vi "Save File DOE File Setup.vi"(0 "Filepath In":T10, 2 "Washer Controls In":T12={"Test Fixture Hardware"={"Power "={"Yokogawa"={"WT210"={"Sample Rate (1: 0.25s)"=1, "A Range (12: 20A)"=12, "V Range (6: 600V)"=4, "Power VISA Yokogawa WT210"="WT210"}, "WT500"={"Power VISA Yokogawa WT500"="WT500", "V Range (8: 1000V)"=0, "I Range (7: 40A)"=0, "Update Rate (3: 500ms)"=2}, "WT310_2"={"Sample Rate (1: 0.25s)"=1, "A Range (12: 20A)"=11, "V Range (6: 600V)"=4, "Power VISA Yokogawa WT310_2"="WT310_2"}, "WT310_3"={"Sample Rate (1: 0.25s)"=1, "A Range (12: 20A)"=11, "V Range (6: 600V)"=4, "Power VISA Yokogawa WT310_3"="WT310_3"}}, "Aplus"={"Aplus IP Address"="192.168.1.101", "Remote Port"=502, "Instrument"="APLUS", "Instr Driver Revision"="1.03.0053"}, "Power Limits"={"Crest Factor"={"Upper Limit"=1.49, "Lower Limit"=1.34}, "Harmonic Content"={"Uthd"=2.0}, "Voltage"={"% Error"=2.0}, "Stability"={"<1 Watt "={"Wattage"=1.0, "Slope (mW/H)"=10.0}, ">1 Watt"={"1%Power/Hour"=1.0}}}, "Nominal Voltage"=120, "Time Limit (s)"=10800.0, "Power Variation Limit (%)"=50.0, "Power Supply"={"Chroma 61605"="CHROMA", "Use Chroma?"=FALSE}}, "Weight Scale"={"Com Options"={"IND560Scale VISA"="IND560", "IP Address"="192.168.1.50", "Remote Port"=502, "Setra Scale VISA"="MW100", "GSE 350"="GSE350"}, "Select Scale"=""}, "Flow Rates"={"Laurel Cold IP Address"="", "Laurel Hot IP Address"="34972A_2", "Hot Water Laurel VISA"="LaurelMeter_Hot", "Cold Water Laurel VISA"="LaurelMeter_Cold", "Remote Port"=0, "Laurel Communication Type"="", "Meters To Collect (Hot Cold)"="", "HOT Laurel Reference"=refnum, "COLD Laurel Reference"=refnum}, "Analog Data"={"Agilent"={"Agilent 34972_1"="34972A_1", "Agilent 34972_2"="34972A_2", "Agilent 34972_3"="34972A_3", "Agilent 34972_4"="34972A_4", "Agilent 34972_5"="34972A_5", "Agilent 34972_6"="34972A_6", "Agilent Gain"=0.0, "TC Type (K,J,T)"="", "Instrument IDN?"="", "TC Channels-List"="", "Analog Channels-List"="", "Agilent Cluster Array"=[], "TC Channels-List 2"="", "Analog Channels-List 2"=""}, "Yokogawa"={"MW100"="MW100", "Intellifaucet"=FALSE}, "Select Analog"="", "TC Coefficients"={"TC Coefficients 1"=[], "TC Coefficients 2"=[], "TC Coefficients 3"=[], "TC Coefficients 4"=[], "TC Coefficients 5"=[], "TC Coefficients 6"=[], "TC Coefficients 7"=[]}, "NI Tasks (Dryer DOE)"=["TC Temps-Module 1", "TC Temps-Module 2", "TC Temps-Module 3", "TC Temps-Module 4", "TC Temps-Module 5", "Gas and Temp-Module 6", "AC_DC Events-Module 7"], "Laurel Analog"={"Laurel IP (Water Temp)"="", "Laurel IP (Pressure)"=""}}, "ITHX-Temp Humidity"={"IP Address 1"="", "Remote Port"=0, "IP Address 2"="", "IP Address 3"=""}, "Gas Meter COM Ports"={"Gas Meter 1"="COM3", "Gas Meter 2"="COM4", "Gas Meter 3"="COM5", "Gas Meter 4"="COM6", "Gas Meter 5"="COM7", "Gas Meter 6"="COM8"}, "Barometric Pressure"={"HEISE 901A"="HEISE", "Use Barometer?"=FALSE}}, "GEA2"={"Address"=35, "Source"=228, "Viper/Hawk"=0}, "DOE Capacity Measurments"={"Weight 1"=35.0, "Model Number 1"="", "Temp 1"=0.0, "Serial Number 1"="", "Lab Number 1"="", "Lab Number 2"="", "Serial Number 2"="", "Temp 2"=0.0, "Model Number 2"="", "Weight 2"=0.0, "Lab Number 3"="", "Serial Number 3"="", "Temp 3"=0.0, "Model Number 3"="", "Weight 3"=0.0, "Lab Number 4"="", "Serial Number 4"="", "Temp 4"=0.0, "Model Number 4"="", "Weight 4"=0.0, "Capacity Measurment Output String"=[]}, "Initialize.Washer In"={"Appliance Details"={"FileVersionInfo"={"FileVersion"="", "ProductName"="", "InternalName"="", "CompanyName"="", "LegalCopyright"="", "FileDescription"=""}, "Dishwasher Info"={"Open Cup Weight (gm):"=0.0, "Auto Cup Weight (gm):"=0.0, "Detergent-Dish:"="", "Inlet Temperature-Dish:"="", "Cycle Mode-Dish:"="", "Unit Control-Dish:"="", "Manufacturer-Dish:"=""}, "Washer Info"={"Hot Water Temperature (Fahrenheit):"="", "Cold Water Temperature (Fahrenheit):"="", "Capacity (cu.ft):"=0.0, "Initial Cloth Weight:"=0.0, "Cloth Lot:"=60, "Model Family:"="", "Program Name:"="", "Cycle Selection:"="", "Wash Temperature:"="", "Rinse Temperature:"="", "Load Size:"=""}, "File Name Output Array"=[], "Calibration Output Array"=[], "Appliance Common"={"Engineer:"="", "Model Number:"="", "Serial Number:"="", "Comments:"="", "Station ID:"="", "Technician:"="", "TR Number:"="", "Lab ID:"="", "Voltage:"="", "Water Pressure (PSI):"="", "Test Date:"="", "Computer Name:"="", "IP Address:"="", "Ambient RH:"="", "Frequency:"="", "Build:"="", "Filename:"="", "Test Type:"="", "Load Run #:"=17, "Ambient Temperature (F):"="", "File Path:"=path "", "Cycles Per Year"=0}, "Water Heater"={"Heating Mode:"=""}, "Dryer"={"Heat Setting:"="", "Washer Water Temperature (60 ± 5°F):"=7, "Water Hardness (PPM):"=7, "Dryness Setting:"="", "Dryer Type:"="", "Exhaust:"="", "Drying Cycle:"="", "Load Type:"="", "Nominal Load Weight"="", "Dryer Initial IMC Data"={"Measured IMC (lbs)"=100.0, "Actual Initial RMC (%)"=7.0, "RMC (Desired %)"=5.0, "Bone Dry Wt(lbs)"=60.0, "Tolerance(%)"=0.0, "Actual Final RMC (%)"=7.0, "CEF (lbf/kWh)"=0.0, "Minimum Weight (lbf)"=0.0, "Average Weight (lbf)"=0.0, "Maximum Weight (lbf)"=0.0, "Measured IMC In Range?"=FALSE, "Moisture Reduction Factor"=55.5, "Field Use Factor"=1.04, "Empty Dryer Cold Weigth"=0.0, "Energy Standard"=enum."D2-Automatic Dryer", "Weight Cloth (lbs)"=0.0, "Relative Moisture Content (%)"=0.0, "Relative Moisture Content - Avg (%)"=0.0}}}, "Display Data (RLT)"={"Status Color"=0, "Serial Number Display"="", "Cycle Count Display"=0, "Station Label Display"="", "Current Run Start Time Display"=0.0, "Board ID Display"="", "RPM Display"=0, "Current Display"=0.0, "Current Path Display"=path "", "Saving Display"=FALSE, "Unit Type Display"=enum."", "Total Time On Display"=0.0, "UI Button"=FALSE}}} {"Initialize.Washer In"."Display Data (RLT)"."Current Display" format="%.2f"; "Initialize.Washer In"."Display Data (RLT)"."Cycle Count Display" format="%04d"; "Initialize.Washer In"."Appliance Details"."Dryer"."Dryer Initial IMC Data"."Maximum Weight (lbf)" format="%03_6g"; "Initialize.Washer In"."Appliance Details"."Dryer"."Dryer Initial IMC Data"."Average Weight (lbf)" format="%03_6g"; "Initialize.Washer In"."Appliance Details"."Dryer"."Dryer Initial IMC Data"."Minimum Weight (lbf)" format="%03_6g"; "Initialize.Washer In"."Appliance Details"."Dryer"."Dryer Initial IMC Data"."CEF (lbf/kWh)" format="%03_6g"; "Initialize.Washer In"."Appliance Details"."Dryer"."Dryer Initial IMC Data"."Actual Final RMC (%)" format="%03_6g"; "Initialize.Washer In"."Appliance Details"."Dryer"."Dryer Initial IMC Data"."Tolerance(%)" format="%0#_6g"; "Initialize.Washer In"."Appliance Details"."Dryer"."Dryer Initial IMC Data"."Bone Dry Wt(lbs)" format="%03_6g"; "Initialize.Washer In"."Appliance Details"."Dryer"."Dryer Initial IMC Data"."RMC (Desired %)" format="%0#_6g"; "Initialize.Washer In"."Appliance Details"."Dryer"."Dryer Initial IMC Data"."Actual Initial RMC (%)" format="%03_6g"; "Initialize.Washer In"."Appliance Details"."Dryer"."Dryer Initial IMC Data"."Measured IMC (lbs)" format="%0#_6g"; "GEA2"."Address" format="%x"; "GEA2"."Source" format="%x"; "GEA2"."Viper/Hawk" items=["Viper", "Hawk"]; "Test Fixture Hardware"."Power"."Yokogawa"."WT310_3"."V Range (6: 600V)" items=["Auto", "15V", "30V", "60V", "150V", "300V", "600V"]; "Test Fixture Hardware"."Power"."Yokogawa"."WT310_3"."A Range (12: 20A)" items=["Auto", "5mA", "10mA", "20mA", "50mA", "100mA", "200mA", "0.5A", "1A", "2A", "5A", "10A", "20A", "50mV", "100mV", "200mV", "2.5V", "5V", "10V"]; "Test Fixture Hardware"."Power"."Yokogawa"."WT310_3"."Sample Rate (1: 0.25s)" items=["0.1s", "0.25s", "0.5s", "1s", "2s", "5s"]; "Test Fixture Hardware"."Power"."Yokogawa"."WT310_2"."V Range (6: 600V)" items=["Auto", "15V", "30V", "60V", "150V", "300V", "600V"]; "Test Fixture Hardware"."Power"."Yokogawa"."WT310_2"."A Range (12: 20A)" items=["Auto", "5mA", "10mA", "20mA", "50mA", "100mA", "200mA", "0.5A", "1A", "2A", "5A", "10A", "20A", "50mV", "100mV", "200mV", "2.5V", "5V", "10V"]; "Test Fixture Hardware"."Power"."Yokogawa"."WT310_2"."Sample Rate (1: 0.25s)" items=["0.1s", "0.25s", "0.5s", "1s", "2s", "5s"]; "Test Fixture Hardware"."Power"."Yokogawa"."WT500"."Update Rate (3: 500ms)" items=["-", "100ms", "200ms", "500ms", "1s", "2s", "5s"]; "Test Fixture Hardware"."Power"."Yokogawa"."WT500"."I Range (7: 40A)" items=["AUTO", "500 mA", "1 A", "2 A", "5 A", "10 A", "20 A", "40 A", "S-AUTO", "50 mV", "100 mV", "200 mV", "500 mV", "1 V", "2 V", "5 V", "10 V", "250 mA", "500 mA", "1 A", "2.5 A", "5 A", "10 A", "20 A", "25 mV", "50 mV", "100 mV", "250 mV", "500 mV", "1 V", "2.5 V", "5 V"]; "Test Fixture Hardware"."Power"."Yokogawa"."WT500"."V Range (8: 1000V)" items=["AUTO", "15", "30", "60", "100", "150", "300", "600", "1000", "7.5", "15", "30", "50", "75", "150", "300", "500"]; "Test Fixture Hardware"."Power"."Yokogawa"."WT210"."V Range (6: 600V)" items=["Auto", "15V", "30V", "60V", "150V", "300V", "600V"]; "Test Fixture Hardware"."Power"."Yokogawa"."WT210"."A Range (12: 20A)" items=["Auto", "5mA", "10mA", "20mA", "50mA", "100mA", "200mA", "0.5A", "1A", "2A", "5A", "10A", "20A", "50mV", "100mV", "200mV", "2.5V", "5V", "10V"]; "Test Fixture Hardware"."Power"."Yokogawa"."WT210"."Sample Rate (1: 0.25s)" items=["0.1s", "0.25s", "0.5s", "1s", "2s", "5s"]}, 3 "Station ID:":string(combo), 5 "error in (no error)":errorcluster, 6 "Config State":T8, 8 "LV Program":T9=enum."DOE Stand") -> (14 "Washer Controls Out":T12={"Test Fixture Hardware"={"Power "={"Yokogawa"={"WT210"={"Sample Rate (1: 0.25s)"=1, "A Range (12: 20A)"=12, "V Range (6: 600V)"=4, "Power VISA Yokogawa WT210"="WT210"}, "WT500"={"Power VISA Yokogawa WT500"="WT500", "V Range (8: 1000V)"=0, "I Range (7: 40A)"=0, "Update Rate (3: 500ms)"=2}, "WT310_2"={"Sample Rate (1: 0.25s)"=1, "A Range (12: 20A)"=11, "V Range (6: 600V)"=4, "Power VISA Yokogawa WT310_2"="WT310_2"}, "WT310_3"={"Sample Rate (1: 0.25s)"=1, "A Range (12: 20A)"=11, "V Range (6: 600V)"=4, "Power VISA Yokogawa WT310_3"="WT310_3"}}, "Aplus"={"Aplus IP Address"="192.168.1.101", "Remote Port"=502, "Instrument"="APLUS", "Instr Driver Revision"="1.03.0053"}, "Power Limits"={"Crest Factor"={"Upper Limit"=1.49, "Lower Limit"=1.34}, "Harmonic Content"={"Uthd"=2.0}, "Voltage"={"% Error"=2.0}, "Stability"={"<1 Watt "={"Wattage"=1.0, "Slope (mW/H)"=10.0}, ">1 Watt"={"1%Power/Hour"=1.0}}}, "Nominal Voltage"=120, "Time Limit (s)"=10800.0, "Power Variation Limit (%)"=50.0, "Power Supply"={"Chroma 61605"="CHROMA", "Use Chroma?"=FALSE}}, "Weight Scale"={"Com Options"={"IND560Scale VISA"="IND560", "IP Address"="192.168.1.50", "Remote Port"=502, "Setra Scale VISA"="SETRA", "GSE 350"="GSE350"}, "Select Scale"=""}, "Flow Rates"={"Laurel Cold IP Address"="", "Laurel Hot IP Address"="", "Hot Water Laurel VISA"="34972A_3", "Cold Water Laurel VISA"="MW100", "Remote Port"=0, "Laurel Communication Type"="", "Meters To Collect (Hot Cold)"="", "HOT Laurel Reference"=refnum, "COLD Laurel Reference"=refnum}, "Analog Data"={"Agilent"={"Agilent 34972_1"="34972A_1", "Agilent 34972_2"="34972A_2", "Agilent 34972_3"="34972A_3", "Agilent 34972_4"="34972A_3", "Agilent 34972_5"="34972A_3", "Agilent 34972_6"="34972A_3", "Agilent Gain"=0.0, "TC Type (K,J,T)"="", "Instrument IDN?"="", "TC Channels-List"="", "Analog Channels-List"="", "Agilent Cluster Array"=[], "TC Channels-List 2"="", "Analog Channels-List 2"=""}, "Yokogawa"={"MW100"="MW100", "Intellifaucet"=FALSE}, "Select Analog"="", "TC Coefficients"={"TC Coefficients 1"=[], "TC Coefficients 2"=[], "TC Coefficients 3"=[], "TC Coefficients 4"=[], "TC Coefficients 5"=[], "TC Coefficients 6"=[], "TC Coefficients 7"=[]}, "NI Tasks (Dryer DOE)"=["TC Temps-Module 1", "TC Temps-Module 2", "TC Temps-Module 3", "TC Temps-Module 4", "TC Temps-Module 5", "Gas and Temp-Module 6", "AC_DC Events-Module 7"], "Laurel Analog"={"Laurel IP (Water Temp)"="", "Laurel IP (Pressure)"=""}}, "ITHX-Temp Humidity"={"IP Address 1"="", "Remote Port"=0, "IP Address 2"="", "IP Address 3"=""}, "Gas Meter COM Ports"={"Gas Meter 1"="COM3", "Gas Meter 2"="COM4", "Gas Meter 3"="COM5", "Gas Meter 4"="COM6", "Gas Meter 5"="COM7", "Gas Meter 6"="COM8"}, "Barometric Pressure"={"HEISE 901A"="HEISE", "Use Barometer?"=FALSE}}, "GEA2"={"Address"=35, "Source"=228, "Viper/Hawk"=0}, "DOE Capacity Measurments"={"Weight 1"=35.0, "Model Number 1"="", "Temp 1"=0.0, "Serial Number 1"="", "Lab Number 1"="", "Lab Number 2"="", "Serial Number 2"="", "Temp 2"=0.0, "Model Number 2"="", "Weight 2"=0.0, "Lab Number 3"="", "Serial Number 3"="", "Temp 3"=0.0, "Model Number 3"="", "Weight 3"=0.0, "Lab Number 4"="", "Serial Number 4"="", "Temp 4"=0.0, "Model Number 4"="", "Weight 4"=0.0, "Capacity Measurment Output String"=[]}, "Initialize.Washer In"={"Appliance Details"={"FileVersionInfo"={"FileVersion"="", "ProductName"="", "InternalName"="", "CompanyName"="", "LegalCopyright"="", "FileDescription"=""}, "Dishwasher Info"={"Open Cup Weight (gm):"=0.0, "Auto Cup Weight (gm):"=0.0, "Detergent-Dish:"="", "Inlet Temperature-Dish:"="", "Cycle Mode-Dish:"="", "Unit Control-Dish:"="", "Manufacturer-Dish:"=""}, "Washer Info"={"Hot Water Temperature (Fahrenheit):"="", "Cold Water Temperature (Fahrenheit):"="", "Capacity (cu.ft):"=0.0, "Initial Cloth Weight:"=0.0, "Cloth Lot:"=60, "Model Family:"="", "Program Name:"="", "Cycle Selection:"="", "Wash Temperature:"="", "Rinse Temperature:"="", "Load Size:"=""}, "File Name Output Array"=[], "Calibration Output Array"=[], "Appliance Common"={"Engineer:"="", "Model Number:"="", "Serial Number:"="", "Comments:"="", "Station ID:"="", "Technician:"="", "TR Number:"="", "Lab ID:"="", "Voltage:"="", "Water Pressure (PSI):"="", "Test Date:"="", "Computer Name:"="", "IP Address:"="", "Ambient RH:"="", "Frequency:"="", "Build:"="", "Filename:"="", "Test Type:"="", "Load Run #:"=17, "Ambient Temperature (F):"="", "File Path:"=path "", "Cycles Per Year"=0}, "Water Heater"={"Heating Mode:"=""}, "Dryer"={"Heat Setting:"="", "Washer Water Temperature (60 ± 5°F):"=7, "Water Hardness (PPM):"=7, "Dryness Setting:"="", "Dryer Type:"="", "Exhaust:"="", "Drying Cycle:"="", "Load Type:"="", "Nominal Load Weight"="", "Dryer Initial IMC Data"={"Measured IMC (lbs)"=100.0, "Actual Initial RMC (%)"=7.0, "RMC (Desired %)"=5.0, "Bone Dry Wt(lbs)"=60.0, "Tolerance(%)"=0.0, "Actual Final RMC (%)"=7.0, "CEF (lbf/kWh)"=0.0, "Minimum Weight (lbf)"=0.0, "Average Weight (lbf)"=0.0, "Maximum Weight (lbf)"=0.0, "Measured IMC In Range?"=FALSE, "Moisture Reduction Factor"=55.5, "Field Use Factor"=1.04, "Empty Dryer Cold Weigth"=0.0, "Energy Standard"=enum."D2-Automatic Dryer", "Weight Cloth (lbs)"=0.0, "Relative Moisture Content (%)"=0.0, "Relative Moisture Content - Avg (%)"=0.0}}}, "Display Data (RLT)"={"Status Color"=0, "Serial Number Display"="", "Cycle Count Display"=0, "Station Label Display"="", "Current Run Start Time Display"=0.0, "Board ID Display"="", "RPM Display"=0, "Current Display"=0.0, "Current Path Display"=path "", "Saving Display"=FALSE, "Unit Type Display"=enum."", "Total Time On Display"=0.0, "UI Button"=FALSE}}} {"Initialize.Washer In"."Display Data (RLT)"."Current Display" format="%.2f"; "Initialize.Washer In"."Display Data (RLT)"."Cycle Count Display" format="%04d"; "Initialize.Washer In"."Appliance Details"."Dryer"."Dryer Initial IMC Data"."Maximum Weight (lbf)" format="%03_6g"; "Initialize.Washer In"."Appliance Details"."Dryer"."Dryer Initial IMC Data"."Average Weight (lbf)" format="%03_6g"; "Initialize.Washer In"."Appliance Details"."Dryer"."Dryer Initial IMC Data"."Minimum Weight (lbf)" format="%03_6g"; "Initialize.Washer In"."Appliance Details"."Dryer"."Dryer Initial IMC Data"."CEF (lbf/kWh)" format="%03_6g"; "Initialize.Washer In"."Appliance Details"."Dryer"."Dryer Initial IMC Data"."Actual Final RMC (%)" format="%03_6g"; "Initialize.Washer In"."Appliance Details"."Dryer"."Dryer Initial IMC Data"."Tolerance(%)" format="%0#_6g"; "Initialize.Washer In"."Appliance Details"."Dryer"."Dryer Initial IMC Data"."Bone Dry Wt(lbs)" format="%03_6g"; "Initialize.Washer In"."Appliance Details"."Dryer"."Dryer Initial IMC Data"."RMC (Desired %)" format="%0#_6g"; "Initialize.Washer In"."Appliance Details"."Dryer"."Dryer Initial IMC Data"."Actual Initial RMC (%)" format="%03_6g"; "Initialize.Washer In"."Appliance Details"."Dryer"."Dryer Initial IMC Data"."Measured IMC (lbs)" format="%0#_6g"; "GEA2"."Address" format="%x"; "GEA2"."Source" format="%x"; "GEA2"."Viper/Hawk" items=["Viper", "Hawk"]; "Test Fixture Hardware"."Power"."Yokogawa"."WT310_3"."V Range (6: 600V)" items=["Auto", "15V", "30V", "60V", "150V", "300V", "600V"]; "Test Fixture Hardware"."Power"."Yokogawa"."WT310_3"."A Range (12: 20A)" items=["Auto", "5mA", "10mA", "20mA", "50mA", "100mA", "200mA", "0.5A", "1A", "2A", "5A", "10A", "20A", "50mV", "100mV", "200mV", "2.5V", "5V", "10V"]; "Test Fixture Hardware"."Power"."Yokogawa"."WT310_3"."Sample Rate (1: 0.25s)" items=["0.1s", "0.25s", "0.5s", "1s", "2s", "5s"]; "Test Fixture Hardware"."Power"."Yokogawa"."WT310_2"."V Range (6: 600V)" items=["Auto", "15V", "30V", "60V", "150V", "300V", "600V"]; "Test Fixture Hardware"."Power"."Yokogawa"."WT310_2"."A Range (12: 20A)" items=["Auto", "5mA", "10mA", "20mA", "50mA", "100mA", "200mA", "0.5A", "1A", "2A", "5A", "10A", "20A", "50mV", "100mV", "200mV", "2.5V", "5V", "10V"]; "Test Fixture Hardware"."Power"."Yokogawa"."WT310_2"."Sample Rate (1: 0.25s)" items=["0.1s", "0.25s", "0.5s", "1s", "2s", "5s"]; "Test Fixture Hardware"."Power"."Yokogawa"."WT500"."Update Rate (3: 500ms)" items=["-", "100ms", "200ms", "500ms", "1s", "2s", "5s"]; "Test Fixture Hardware"."Power"."Yokogawa"."WT500"."I Range (7: 40A)" items=["AUTO", "500 mA", "1 A", "2 A", "5 A", "10 A", "20 A", "40 A", "S-AUTO", "50 mV", "100 mV", "200 mV", "500 mV", "1 V", "2 V", "5 V", "10 V", "250 mA", "500 mA", "1 A", "2.5 A", "5 A", "10 A", "20 A", "25 mV", "50 mV", "100 mV", "250 mV", "500 mV", "1 V", "2.5 V", "5 V"]; "Test Fixture Hardware"."Power"."Yokogawa"."WT500"."V Range (8: 1000V)" items=["AUTO", "15", "30", "60", "100", "150", "300", "600", "1000", "7.5", "15", "30", "50", "75", "150", "300", "500"]; "Test Fixture Hardware"."Power"."Yokogawa"."WT210"."V Range (6: 600V)" items=["Auto", "15V", "30V", "60V", "150V", "300V", "600V"]; "Test Fixture Hardware"."Power"."Yokogawa"."WT210"."A Range (12: 20A)" items=["Auto", "5mA", "10mA", "20mA", "50mA", "100mA", "200mA", "0.5A", "1A", "2A", "5A", "10A", "20A", "50mV", "100mV", "200mV", "2.5V", "5V", "10V"]; "Test Fixture Hardware"."Power"."Yokogawa"."WT210"."Sample Rate (1: 0.25s)" items=["0.1s", "0.25s", "0.5s", "1s", "2s", "5s"]}, 16 "Filepath Out":T10, 19 "error out":errorcluster)   [LabVIEW 2018, in "File Setup.lvlib"]
uses:
  File Setup.lvlib
  Custom Pallet Controls/Custom Pallet String.ctl
  Custom Pallet Controls/Custom Pallet Forward.ctl
  Type Definition/Save File DOE LabView Program.ctl
  Type Definition/Save File DOE File Path Control.ctl
  Type Definition/Save File DOE Data Save Filepaths.ctl
  Type Definition/Save File DOE Configuration State.ctl
  Type Definition/Save File HEWH Heating Control Mode.ctl
  Washer DOE/Type Definitions/DOE Main Control.ctl
  Washer DOE/Type Definitions/DOE Test Fixture Hardware.ctl
  Type Definitions/UTILITY Power Inputs Control.ctl
  Drivers/IND560 Scale Monitor/Type Definitions/IND560 Configuration.ctl
  Hybrid Water Heater/Type Definitions/HEWH Agilent Cluster.ctl
  Type Definitions/UTILITY TC Coefficients.ctl
  Drivers/Omega FMA-1600A Series Gas Flow Meter/Type Definitions/FMA1600A COM Ports.ctl
  Washer DOE/Configuration/GEA2.ctl
  Washer DOE/Type Definitions/DOE Capacity Measurments.ctl
  Public/Type Definitions/Save File Washer.ctl
  Type Definition/Save File DISH Dishwasher Details.ctl
  <vilib>/Platform/fileVersionInfo.llb/FileVersionInformation.ctl
  Washer DOE/Type Definitions/DOE Appliance Common.ctl
  Type Definition/DPT IMC Data.ctl
  Washer DOE/Type Definitions/DOE Dryer Standard.ctl
  Public/Type Definitions/Save File Appliance Display.ctl
  Public/Type Definitions/Save File Unit Type.ctl
  GEA2 Commands/HEWH/Type Definitions/GEA2 Commands.ctl
  Type Definition/Save File Drop Down Controls.ctl
  <vilib>/Utility/file.llb/Write To Spreadsheet File (string).vi
  LabVIEW GEA2 Toolkit v1.0.0.0/library/GEA2_Toolkit.lvlib
  Save File.lvlib
panel:
  in  "Read Previous":bool
  in  "Comments:":string
  in  "Program Tab":T1(tab)
  in  "Remove Button 23":bool
  in  "Add Button 23":bool
  in  "Ambient Temperature (F):":string(combo)
  in  "Get Serial Number":bool
  in  "Get Model Number":bool
  in  "Remove Button 17":bool
  in  "Add Button 17":bool
  in  "Lab ID:":string(combo)
  in  "Remove Button 1":bool
  in  "Add Button 1":bool
  in  "Remove Button 2":bool
  in  "Add Button 2":bool
  in  "Technician:":string(combo)
  in  "Remove Button 3":bool
  in  "Add Button 3":bool
  in  "Water Pressure (PSI):":string(combo)
  in  "Remove Button 4":bool
  in  "Add Button 4":bool
  in  "Ambient RH:":string(combo)
  in  "Remove Button 5":bool
  in  "Add Button 5":bool
  in  "Supply Voltage:":string(combo)
  in  "Remove Button 6":bool
  in  "Add Button 6":bool
  in  "Frequency:":string(combo)
  in  "Remove Button 7":bool
  in  "Add Button 7":bool
  in  "Build:":string(combo)
  in  "TR Number:":string(combo)
  in  "Remove Button 16":bool
  in  "Add Button 16":bool
  in  "Remove Button 12":bool
  in  "Add Button 12":bool
  in  "Test Type:":string(combo)
  in  "Load Run #:":i32
  in  "Model:":T2
  in  "Serial Number:":T2
  in  "Engineer:":T2
  in  "Cycles Per Year":u32=283
  in  "Remove Button 21":bool
  in  "Add Button 21":bool
  in  "Cycle Selection":string(combo)
  in  "Remove Button 18":bool
  in  "Add Button 18":bool
  in  "Wash Temperature":string(combo)
  in  "Remove Button 19":bool
  in  "Add Button 19":bool
  in  "Rinse Temperature":string(combo)
  in  "Remove Button 20":bool
  in  "Add Button 20":bool
  in  "Load Size":string(combo)
  in  "Remove Button 9":bool
  in  "Add Button 9":bool
  in  "Cold Water Temperature (Fahrenheit)":string(combo)
  in  "Program Name":string(combo)
  in  "Model Family":string(combo)
  in  "Cloth Lot:":i32
  in  "Initial Cloth Weight:":dbl
  in  "Capacity (cu.ft)":dbl
  in  "Hot Water Temperature (Fahrenheit)":string(combo)
  in  "Remove Button 8":bool
  in  "Add Button 8":bool
  in  "Unit Type Display":T3
  in  "Remove Button 15":bool
  in  "Add Button 15":bool
  in  "Detergent-Dish:":string(combo)
  in  "Remove Button 14":bool
  in  "Add Button 14":bool
  in  "Inlet Temperature-Dish:":string(combo)
  in  "Remove Button 13":bool
  in  "Add Button 13":bool
  in  "Cycle Mode-Dish:":string(combo)
  in  "Remove Button 11":bool
  in  "Add Button 11":bool
  in  "Unit Control-Dish:":string(combo)
  in  "Manufacturer-Dish:":string(combo)
  in  "Remove Button 10":bool
  in  "Add Button 10":bool
  in  "Auto Cup Weight (gm):":dbl
  in  "Open Cup Weight (gm):":dbl
  in  "Heating Mode":T4
  in  "Remove Button 22":bool
  in  "Add Button 22":bool
  in  "Energy Standard":T5
  in  "Field Use Factor":dbl
  in  "Moisture Reduction Factor":dbl=55.5
  in  "Get Data":bool
  out "In Range?":string
  in  "Measured Weight (lbf)":dbl format="%#_5g"
  out "Measured Conent (%)":dbl format="%#_5g"
  out "Maximum Weight (lbf)":dbl format="%#_5g"
  out "Average Weight (lbf)":dbl format="%#_5g"
  out "Minimum Weight (lbf)":dbl format="%#_5g"
  in  "Tolerance (%)":dbl=0.33 format="%#_5g"
  in  "Relative Moisture (%)":dbl min=0.0 max=100.0 format="%#_5g"
  in  "Bone Dry Weight (lbf)":dbl min=0.0 max=100.0 format="%#_5g"
  in  "Remove Button 30":bool
  in  "Remove Button 29":bool
  in  "Remove Button 28":bool
  in  "Remove Button 27":bool
  in  "Remove Button 26":bool
  in  "Remove Button 25":bool
  in  "Remove Button 24":bool
  in  "Add Button 30":bool
  in  "Add Button 29":bool
  in  "Add Button 28":bool
  in  "Add Button 27":bool
  in  "Add Button 26":bool
  in  "Add Button 25":bool
  in  "Add Button 24":bool
  in  "Load Type:":string(combo)
  in  "Nominal Load Weight (lbs):":string(combo)
  in  "Dryness Setting:":string(combo)
  in  "Heat Setting:":string(combo)
  in  "Get Weigth":bool
  in  "Cold Dryer Weigth":dbl
  in  "Drying Cycle:":string(combo)
  in  "Exhaust:":string(combo)
  in  "Water Hardness (PPM):":u16=17
  in  "Washer Water Temperature (60 ± 5°F):":u16=60
  in  "Dryer Type:":string(combo)
  in  "Save As Default":bool
  in  "Initialize Default":bool
  out "Description":string="File Name Setup"
  in  "OK":T6
  in  "Tab Control":T7(tab)
  out "Move Past Main Tab":bool
  out "Unhandled Error":errorcluster
  in  "Debug":bool
  out "States":string[](array[string])
  # "Field Use Factor = 1.04 (Automatic Termination)\nField Use Factor = 1.18 (Only Timer Dryers) \nD1 = [53.5/(Ww-Wd)] × Ett × field use"
  # "Field Use Factor = 1.18 (Only Timer Dryers) \nD2 = [55.5/(Ww- Wd)] × Et × field use (Timer Dryer Only)\nD2 = Et (Automatic Termination)"
  # "Target Values"
  # "Weight Range (lbf)"
  # "Actual Content"
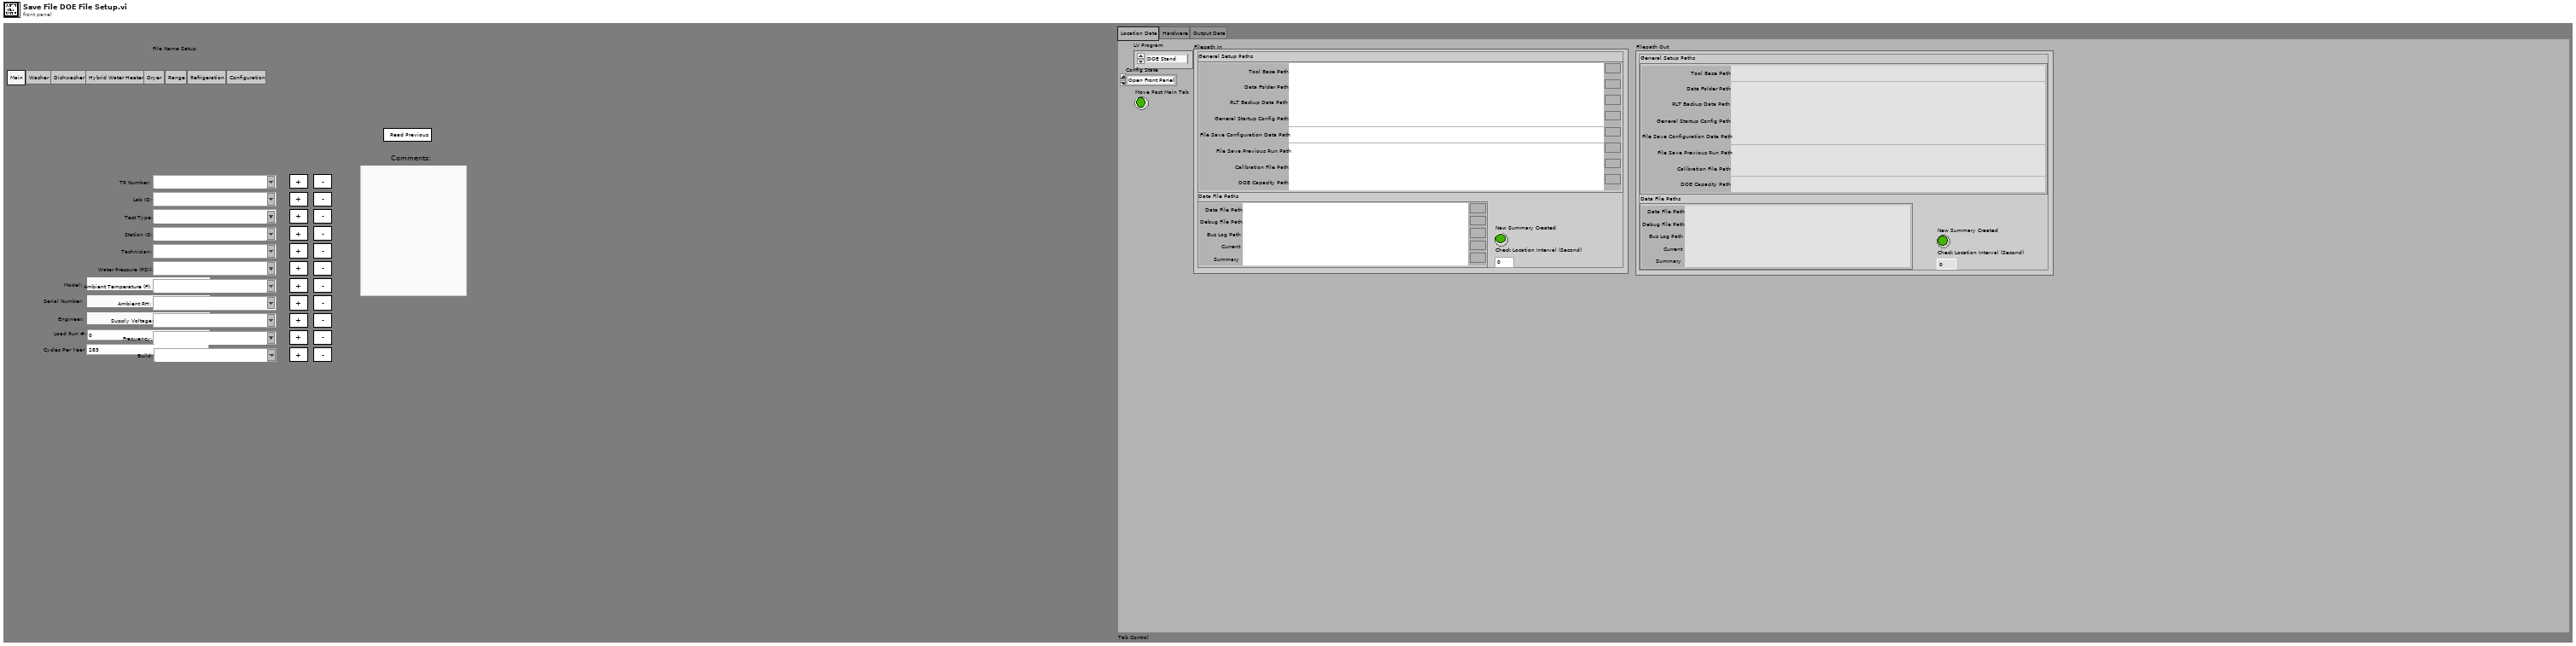
[diagram p1: front panel]
types:
  T1 = enum32{"Main", "Washer", "Dishwasher", "Hybrid Water Heater", "Dryer", "Range", "Refrigeration", "Configuration"}
  T2 = typedef "Custom Pallet String.ctl" = string
  T3 = typedef "Save File.lvlib/Save File Unit Type.ctl" = enum32{"", "Viper", "Hawk", "2015"}
  T4 = typedef "File Setup.lvlib/Save File HEWH Heating Control Mode.ctl" = string
  T5 = typedef "DOE Dryer Standard.ctl" = enum16{"D2-Automatic Dryer", "D2-Timer Dryer", "D1-Automatic Dryer", "D1-Timer Dryer", "Other"}
  T6 = typedef "Custom Pallet Forward.ctl" = bool
  T7 = enum32{"Location Data", "Hardware", "Output Data"}
  T8 = typedef "File Setup.lvlib/Save File DOE Configuration State.ctl" = enum16{"Open Front Panel", "Load Config"}
  T9 = typedef "File Setup.lvlib/Save File DOE LabView Program.ctl" = enum16{"No Name Found", "DOE Stand", "Dishwasher Kitchen", "Portable Stand", "HEWH", "Dryer", "Dryer WILT", "HCC", "PRAT", "HEWH RLT", "Refrigeration"}
  T10 = typedef "File Setup.lvlib/Save File DOE File Path Control.ctl" = cluster{"General Setup Paths":cluster{"Calibration File Path":path, "DOE Capacity Path":path, "Data Folder Path":path, "RLT Backup Data Path":path, "Tool Base Path":path, "General Startup Config Path":path, "File Save Previous Run Path":path, "File Save Configuration Data Path":path}, "Data File Paths":T11, "New Summary Created":bool, "Check Location Interval (Second)":i32}
  T11 = typedef "File Setup.lvlib/Save File DOE Data Save Filepaths.ctl" = cluster{"Data File Path":path, "Debug File Path":path, "Bus Log Path":path, "Current":path, "Summary":path}
  T12 = typedef "DOE Main Control.ctl" = cluster{"Test Fixture Hardware":T13, "GEA2":T19, "DOE Capacity Measurments":T20, "Initialize.Washer In":T21}
  T13 = typedef "DOE Test Fixture Hardware.ctl" = cluster{"Power ":T14, "Weight Scale":cluster{"Com Options":T15, "Select Scale":string}, "Flow Rates":cluster{"Laurel Cold IP Address":string, "Laurel Hot IP Address":string, "Hot Water Laurel VISA":refnum<visa-resource-name>, "Cold Water Laurel VISA":refnum<visa-resource-name>, "Remote Port":u16, "Laurel Communication Type":string, "Meters To Collect (Hot Cold)":string, "HOT Laurel Reference":refnum<k5>, "COLD Laurel Reference":refnum<k5>}, "Analog Data":cluster{"Agilent":cluster{"Agilent 34972_1":refnum<visa-resource-name>, "Agilent 34972_2":refnum<visa-resource-name>, "Agilent 34972_3":refnum<visa-resource-name>, "Agilent 34972_4":refnum<visa-resource-name>, "Agilent 34972_5":refnum<visa-resource-name>, "Agilent 34972_6":refnum<visa-resource-name>, "Agilent Gain":dbl, "TC Type (K,J,T)":string, "Instrument IDN?":string, "TC Channels-List":string, "Analog Channels-List":string, "Agilent Cluster Array":T16[], "TC Channels-List 2":string, "Analog Channels-List 2":string}, "Yokogawa":cluster{"MW100":refnum<visa-resource-name>, "Intellifaucet":bool}, "Select Analog":string, "TC Coefficients":T17, "NI Tasks (Dryer DOE)":refnum<k21>[], "Laurel Analog":cluster{"Laurel IP (Water Temp)":string, "Laurel IP (Pressure)":string}}, "ITHX-Temp Humidity":cluster{"IP Address 1":string, "Remote Port":u16, "IP Address 2":string, "IP Address 3":string}, "Gas Meter COM Ports":T18, "Barometric Pressure":cluster{"HEISE 901A":refnum<visa-resource-name>, "Use Barometer?":bool}}
  T14 = typedef "UTILITY Power Inputs Control.ctl" = cluster{"Yokogawa":cluster{"WT210":cluster{"Sample Rate (1: 0.25s)":i32, "A Range (12: 20A)":i32, "V Range (6: 600V)":i32, "Power VISA Yokogawa WT210":refnum<visa-resource-name>}, "WT500":cluster{"Power VISA Yokogawa WT500":refnum<visa-resource-name>, "V Range (8: 1000V)":i32, "I Range (7: 40A)":i32, "Update Rate (3: 500ms)":i32}, "WT310_2":cluster{"Sample Rate (1: 0.25s)":i32, "A Range (12: 20A)":i32, "V Range (6: 600V)":i32, "Power VISA Yokogawa WT310_2":refnum<visa-resource-name>}, "WT310_3":cluster{"Sample Rate (1: 0.25s)":i32, "A Range (12: 20A)":i32, "V Range (6: 600V)":i32, "Power VISA Yokogawa WT310_3":refnum<visa-resource-name>}}, "Aplus":cluster{"Aplus IP Address":string, "Remote Port":i32, "Instrument":string, "Instr Driver Revision":string}, "Power Limits":cluster{"Crest Factor":cluster{"Upper Limit":dbl, "Lower Limit":dbl}, "Harmonic Content":cluster{"Uthd":dbl}, "Voltage":cluster{"% Error":dbl}, "Stability":cluster{"<1 Watt ":cluster{"Wattage":dbl, "Slope (mW/H)":dbl}, ">1 Watt":cluster{"1%Power/Hour":dbl}}}, "Nominal Voltage":i32, "Time Limit (s)":dbl, "Power Variation Limit (%)":dbl, "Power Supply":cluster{"Chroma 61605":refnum<visa-resource-name>, "Use Chroma?":bool}}
  T15 = typedef "IND560 Configuration.ctl" = cluster{"IND560Scale VISA":refnum<visa-resource-name>, "IP Address":string, "Remote Port":u16, "Setra Scale VISA":refnum<visa-resource-name>, "GSE 350":refnum<visa-resource-name>}
  T16 = typedef "HEWH Agilent Cluster.ctl" = cluster{"Label":string, "Agilent Channel":string, "Panel ID":string, "Source":string, "Temperature":dbl}
  T17 = typedef "UTILITY TC Coefficients.ctl" = cluster{"TC Coefficients 1":dbl[], "TC Coefficients 2":dbl[], "TC Coefficients 3":dbl[], "TC Coefficients 4":dbl[], "TC Coefficients 5":dbl[], "TC Coefficients 6":dbl[], "TC Coefficients 7":dbl[]}
  T18 = typedef "FMA1600A COM Ports.ctl" = cluster{"Gas Meter 1":refnum<visa-resource-name>, "Gas Meter 2":refnum<visa-resource-name>, "Gas Meter 3":refnum<visa-resource-name>, "Gas Meter 4":refnum<visa-resource-name>, "Gas Meter 5":refnum<visa-resource-name>, "Gas Meter 6":refnum<visa-resource-name>}
  T19 = typedef "GEA2.ctl" = cluster{"Address":u8, "Source":u8, "Viper/Hawk":u8}
  T20 = typedef "DOE Capacity Measurments.ctl" = cluster{"Weight 1":dbl, "Model Number 1":string, "Temp 1":dbl, "Serial Number 1":string, "Lab Number 1":string, "Lab Number 2":string, "Serial Number 2":string, "Temp 2":dbl, "Model Number 2":string, "Weight 2":dbl, "Lab Number 3":string, "Serial Number 3":string, "Temp 3":dbl, "Model Number 3":string, "Weight 3":dbl, "Lab Number 4":string, "Serial Number 4":string, "Temp 4":dbl, "Model Number 4":string, "Weight 4":dbl, "Capacity Measurment Output String":string[][]}
  T21 = typedef "Save File.lvlib/Save File Washer.ctl" = cluster{"Appliance Details":T22, "Display Data (RLT)":T26}
  T22 = typedef "File Setup.lvlib/Save File DISH Dishwasher Details.ctl" = cluster{"FileVersionInfo":T23, "Dishwasher Info":cluster{"Open Cup Weight (gm):":dbl, "Auto Cup Weight (gm):":dbl, "Detergent-Dish:":string, "Inlet Temperature-Dish:":string, "Cycle Mode-Dish:":string, "Unit Control-Dish:":string, "Manufacturer-Dish:":string}, "Washer Info":cluster{"Hot Water Temperature (Fahrenheit):":string, "Cold Water Temperature (Fahrenheit):":string, "Capacity (cu.ft):":dbl, "Initial Cloth Weight:":dbl, "Cloth Lot:":i32, "Model Family:":string, "Program Name:":string, "Cycle Selection:":string, "Wash Temperature:":string, "Rinse Temperature:":string, "Load Size:":string}, "File Name Output Array":string[][], "Calibration Output Array":string[][], "Appliance Common":T24, "Water Heater":cluster{"Heating Mode:":string}, "Dryer":cluster{"Heat Setting:":T2, "Washer Water Temperature (60 ± 5°F):":u16, "Water Hardness (PPM):":u16, "Dryness Setting:":T2, "Dryer Type:":string, "Exhaust:":string, "Drying Cycle:":string, "Load Type:":string, "Nominal Load Weight":string, "Dryer Initial IMC Data":T25}}
  T23 = typedef "FileVersionInformation.ctl" = cluster{"FileVersion":string, "ProductName":string, "InternalName":string, "CompanyName":string, "LegalCopyright":string, "FileDescription":string}
  T24 = typedef "DOE Appliance Common.ctl" = cluster{"Engineer:":string, "Model Number:":string, "Serial Number:":string, "Comments:":string, "Station ID:":string, "Technician:":string, "TR Number:":string, "Lab ID:":string, "Voltage:":string, "Water Pressure (PSI):":string, "Test Date:":string, "Computer Name:":string, "IP Address:":string, "Ambient RH:":string, "Frequency:":string, "Build:":string, "Filename:":string, "Test Type:":string, "Load Run #:":i32, "Ambient Temperature (F):":string, "File Path:":path, "Cycles Per Year":u32}
  T25 = typedef "DPT IMC Data.ctl" = cluster{"Measured IMC (lbs)":dbl, "Actual Initial RMC (%)":dbl, "RMC (Desired %)":dbl, "Bone Dry Wt(lbs)":dbl, "Tolerance(%)":dbl, "Actual Final RMC (%)":dbl, "CEF (lbf/kWh)":dbl, "Minimum Weight (lbf)":dbl, "Average Weight (lbf)":dbl, "Maximum Weight (lbf)":dbl, "Measured IMC In Range?":bool, "Moisture Reduction Factor":dbl, "Field Use Factor":dbl, "Empty Dryer Cold Weigth":dbl, "Energy Standard":T5, "Weight Cloth (lbs)":dbl, "Relative Moisture Content (%)":dbl, "Relative Moisture Content - Avg (%)":dbl}
  T26 = typedef "Save File Appliance Display.ctl" = cluster{"Status Color":u32, "Serial Number Display":string, "Cycle Count Display":i32, "Station Label Display":string, "Current Run Start Time Display":dbl, "Board ID Display":string, "RPM Display":u32, "Current Display":dbl, "Current Path Display":path, "Saving Display":bool, "Unit Type Display":T3, "Total Time On Display":dbl, "UI Button":bool}
  T27 = enum16{"Load Standard", "Remove", "Add", "Update"}
  T28 = enum32{"invalid app kind", "Development System", "Run Time System", "Student Edition", "Embedded LabVIEW", "Evaluation", "Custom"}
  T29 = enum32{"Invalid", "Standard", "Closed", "Hidden", "Minimized", "Maximized"}
  T30 = typedef "GEA2 Commands.ctl" = enum16{"CMD_CANCEL_EEV_POSITION", "CMD_CLEAR_ENERGY_USAGE_CTRS", "CMD_CLEAR_FAULT_COUNTS", "CMD_CLEAR_OVERRIDE_STATUS", "CMD_COMP_OFF", "CMD_COMP_ON", "CMD_DSM_OVERRIDES", "CMD_EEV_POSITION", "CMD_ENTER_EXIT_FCT_MODE", "CMD_ENTER_FACT_MODE", "CMD_HP_RUN_6MIN", "CMD_INITIATE_REMOTE_DSM_OVERRIDE", "CMD_LE_2_SECONDS", "CMD_REFRESH_SERVICE_TIMEOUTS", "CMD_RESET", "CMD_RESET_FILTER_TIMES", "CMD_RESTORE_EEPROM_DEFAULTS", "CMD_RQST_LED_STATUS", "CMD_SET_AMBIENT_THRESH_1", "CMD_SET_AMBIENT_THRESH_2", "CMD_SET_AMBIENT_THRESH_3", "CMD_SET_CURRENTS", "CMD_SET_EEV_DRIVE_LINES", "CMD_SET_EEV_STOP_POSITION", "CMD_SET_LEDS", "CMD_SET_MODEL_NUMBER", "CMD_SET_PID_I_DENOM_OVER_THR", "CMD_SET_PID_I_DENOM_UNDER_THR", "CMD_SET_PID_LOW_SH_TARGET", "CMD_SET_PID_MID_SH_TARGET", "CMD_SET_PID_P_DENOMINATOR", "CMD_SET_SERIAL_NUMBER", "CMD_SET_START_POS_OVER_THR", "CMD_SET_START_POS_UNDER_THR", "CMD_TOGGLE_FAN", "CMD_TOGGLE_LE_SERV", "CMD_TOGGLE_SERVICE_MODE", "CMD_TOGGLE_UE_SERV", "CMD_TURN_ON_OFF_DLB", "CMD_UE_2_SECONDS", "CMD_UPDATE_DSM_LEVEL", "CMD_UPDATE_MODE", "CMD_WRITE_SETPOINTS", "REQ_READ_KEY_STATUS", "REQ_SYSTEM_MODE", "RQST_CURRENT_PID_SH_TARGET", "RQST_DATA_FROM_DATA_FLASH", "RQST_DATA_FROM_MEMORY", "RQST_DSM_OVERRIDE_STATUS", "RQST_HEM_KWH_DATA", "RQST_HYPERTERM_OUTPUT_DATA", "RQST_IDLB_RESISTANCE", "RQST_MODEL_NUMBER", "RQST_MODEL_SELECT_AD_VALUE", "RQST_OTHER_FAULT_COUNTS", "RQST_OVERRIDE_STATUS", "RQST_PID_PARAMETERS", "RQST_READ_PERSONALITY", "RQST_SERIAL_NUMBER", "RQST_SERVICE_ERROR_CODES", "RQST_Software_Version", "RQST_SS_FAULT_COUNTS", "RQST_STATUS_QUERY", "RQST_STD_ELEC_RANGE", "RQST_SUPPORTED_MODES", "RQST_T2_RESISTANCE", "RQST_T3B_RESISTANCE", "RQST_T4_RESISTANCE", "RQST_T5_RESISTANCE", "RQST_TEMP_RANGE", "RQST_VACATION_RANGE", "RQST_WATER_CAPACITY"}
  T31 = typedef "GEA2_Toolkit.lvlib/Data In.ctl" = cluster{"Source":u8, "Destination":u8, "Command":u8, "Message":string}
  T32 = typedef "GEA2_Toolkit.lvlib/Data Out.ctl" = cluster{"Source":u8, "Destination":u8, "Command":u8, "Length":u8, "CRC":u16, "Message":string}
  T33 = typedef "ViperHawk Data.ctl" = cluster{"GEA Diagnostic Data - Washer":T34, "Software Version":T35, "Debug Search Parameters":T36, "Message Count":i32, "Number of Messages":i32, "Partial Message String":string, "Full Message to Save":string, "Board ID":string, "Board Index":i32, "Source Address":u8, "Destination Address":u8, "Data to send":u8[], "ReceivedData":u8[], "Debug/GEA Data":string[], "Command":u8, "GEA2 Reference Out":refnum<k24>, "GEA2 Event Registration":refnum<event-registration>, "Bus Data":string, "GEA Data":string[][], "Network Variable Location":i32, "Water Heater GEA2 Data":T37}
  T34 = typedef "ViperHawk Diagnostic Data.ctl" = cluster{"Speed (RPM)":u32, "Load Size":u32, "Temperature":u32, "Water Pressure":dbl, "Detergent":u32, "Fabric Softener":u32, "Tub Direction":string, "Detergent Valve":bool, "Fabric Softener Valve":bool, "Recirculating Pump":bool, "Drain Valve":bool, "Hot Valve":bool, "Cold Valve":bool, "Lid Closed Status":string, "Lid Lock Status":string, "Error Count":u32, "IGBT Temperature (Deg C)":u32, "Motor Speed":u32, "Latched OOB":u32, "Raw OOB":u32, "Plaster Status":u32, "Inverter Power (W)":u32, "Target Speed(BRPM)":u32, "Latched Agitate Motor Temp (Deg C)":u32, "Current Motor Temp (Deg C)":u32, "Profiler Status":string, "Current Inverter Action":string, "Error Codes":string, "Lid Locked":bool, "Lid Closed":bool, "9E Diagnostic Data":cluster{"Total Cycle Time (Min)":u32, "Total Cycle Count (Current)":u16, "Total Error Count":u16, "Machine Error History":u32, "Washer UI History":u32, "Inverter Error History":u32, "Cycle Storage Limit":u8, "Error Storage Limit":u8, "Cycle Pages Supported":u8, "Error Pages Supported":u8, "Inverter Reset Count":u16}, "9F Diagnostic Data":cluster{"Cycle Buffer Index":string, "Page Number":string, "Total Cycle Count":u32, "Delay Start Time":u32, "Stain Selected":string, "Selected Cycle":u32, "eWash":string, "Soil Level":string, "Temperature":string, "Overnight Ready":string, "Spin Setting":string, "Control Lock Status":string, "Stain Remover":string, "Steam Assist":string, "My Cycle":string, "PreWash":string, "Debug Log Enabled":string, "Rinse":string, "Signal Level":string, "PreSoak":string}}
  T35 = typedef "Save File.lvlib/Save File Software Version.ctl" = cluster{"Critical Major SW Version":string, "Critical Minor SW Version":string, "Major SW Version":string, "Minor SW Version":string, "Parametric Data Ver. Major":string, "Parametric Data Ver. Minor":string, "Diagnostics Data Ver. Major":string, "Diagnostics Data Ver. Minor":string, "Current Personality Setting":string}
  T36 = typedef "ViperHawk Search Control.ctl" = cluster{"Pause":string[], "Run":string[], "EOC":string[], "Error Codes":string[]}
  T37 = typedef "GEA2 Commands WaterHeater GEA2 Data.ctl" = cluster{"GEA2 Label Array":string[], "PID_PARAMETERS":string[][], "SUPPORTED_MODES":string[][], "Button Status":T38, "Status Query":T39, "Service Error Codes":T40, "HEM_KWH_DATA":string[][], "OTHER_FAULT_COUNTS":string[][], "GEA2 Raw Message":string, "Hyperterminal Data":cluster{"Source":u8, "Destination":u8, "Command":u8, "Length":u8, "CRC":u16, "UE - state (1/0 on off)":u8, "LE - state (1/0 on off)":u8, "Comp - state (1/0 on off)":u8, "Fan  - state (1/0 on off)":u8, "Setpoint Deg F":i32, "T2(TankSensor)":dbl, "T3A(EvapIn)":dbl, "T3B(EvapOut)":dbl, "T4(CompressorDischarge)":dbl, "T5(Ambient)":dbl, "Current":dbl, "Voltage (Volts)":u16, "EEV Position (0-480)":u16, "Reason for last heating cycle termination":u16, "Reason Data word 1":string, "Reason Data word 2":string, "Reason Data word 3":string, "Reason Data word 4":string, "SW Debug Data":string, "Flow Events (Bit Encoded)":u16, "Heating Control Mode":u16}, "Extra Data":cluster{"Water Capacity (Gallons)":u32, "Max Vacation Duration Days":u32, "Min Vacation Duration Days":u32, "Max Set Point (Deg F)":u32, "Min Set Point (Deg F)":u32, "T5 Resistance":u32, "T4 Resistance":u32, "T3B Resistance":u32, "T2 Resistance":u32, "STD_ELEC_RANGE":string, "SS_FAULT_COUNTS":string, "SERIAL_NUMBER":string, "READ_PERSONALITY":u8, "RQST_OVERRIDE_STATUS":string, "MODEL_SELECT_AD_VALUE":u32, "MODEL NUMBER":string, "IDLB_RESISTANCE":u32, "DSM Override Status":string, "RQST_DATA_FROM_Memory":string, "RQST_DATA_FROM_DATA_FLASH":string, "RQST_CURRENT_PID_SH_TARGET":u16, "Unit System Mode":string}}
  T38 = typedef "GEA2 Commands Button Status.ctl" = cluster{"Switch 1":bool, "Switch 2":bool, "Switch 3":bool, "Switch 4":bool, "Switch 5":bool, "Switch 6":bool, "Switch 7":bool, "Switch 8":bool, "Switch 9":bool, "Switch 10":bool, "Switch 11":bool, "Switch 12":bool, "Switch 13":bool, "Switch 14":bool, "Switch 15":bool, "Switch 16":bool}
  T39 = typedef "GEA2 Commands Status Query.ctl" = cluster{"Days Remaining (For Std Electric and Vacation)":u8, "Unit Status":string, "Current Tank Temp in Deg F":u8, "Current Setpoint in Deg F":u8, "Filter Status (% used)":u8, "Fallback Status (Fallback heating mode)":string, "Fallback Temp":u8, "\"Set Mode\" Selection":string}
  T40 = typedef "GEA2 Commands Service Error Codes.ctl" = cluster{"Reserved":bool, "Reserved 1":bool, "Reserved 2":bool, "Reserved 3":bool, "Reserved 4":bool, "Reserved 5":bool, "Reserved 6":bool, "Reserved 7":bool, "DataFlash Fail Status":bool, "Stuck Key Fail Status":bool, "Dry Tank Fail Status":bool, "Miswire Fail Status":bool, "Reserved 8":bool, "Reserved 9":bool, "Reserved 10":bool, "Reserved 11":bool, "UE Fail Status":bool, "LE Fail Status":bool, "Filter Fail Status":bool, "T3A Fail Status":bool, "T3B Fail Status":bool, "T4 Fail Status":bool, "T5 Fail Status":bool, "T2 Fail Status":bool, "SS Cond A Status":bool, "SS Cond B Status":bool, "SS Cond C Status":bool, "SS Cond D Status":bool, "SS Cond E Status":bool, "SS Cond F Status":bool, "SS Fan Status":bool, "CMP Fail Status":bool}
  T41 = typedef "File Setup.lvlib/Save File Drop Down Controls.ctl" = cluster{"Manufacturer-Dish (Array):":string[], "Unit Control-Dish (Array):":string[], "Test Type (Array):":string[], "Cycle Mode-Dish(Array): ":string[], "Inlet Temperature (F)-Dish (Array):":string[], "Detergent-Dish (Array):":string[], "Cycle Selection (Array):":string[], "Wash Temperature (Array):":string[], "Rinse Temperature (Array):":string[], "Load Size (Array):":string[], "Water Pressure (PSI) (Array) :":string[], "Ambient RH (Array):":string[], "Supply Voltage (Array):":string[], "Station ID (Array):":string[], "Lab ID (Array):":string[], "TR Number (Array):":string[], "Cold Water Temperature (Fahrenheit) (Array):":string[], "Technician (Array):":string[], "Frequency (Array):":string[], "Build (Array):":string[], "Hot Water Temperature (Fahrenheit) (Array):":string[], "Heating Mode (Array):":string[], "Ambient Temperature (F) (Array):":string[], "Dryer Type (Array):":string[], "Exhaust (Array):":string[], "Drying Cycle (Array):":string[], "Heat Setting (Array):":string[], "Dryness Setting (Array):":string[], "Nominal Load Weigth (lbs) (Array):":string[], "Load Type (Array):":string[]}
  T42 = cluster{"Core":cluster{"Current VI Reference":refnum<vi>, "Close Panel on Exit?":bool}, "Error Flag":bool, "Washer Controls In":T12, "LV Program":T9, "Filepath In":T10, "Drop Down Controls":T41}
  T43 = cluster{"Current VI Reference":refnum<vi>, "Close Panel on Exit?":bool}
  T44 = typedef "File Setup.lvlib/Save File DOE Configuration File.ctl" = cluster{"File Search":string[], "Model Details Header":string[], "Drop Down Controls":T41, "End of Cycle Commands":string[]}
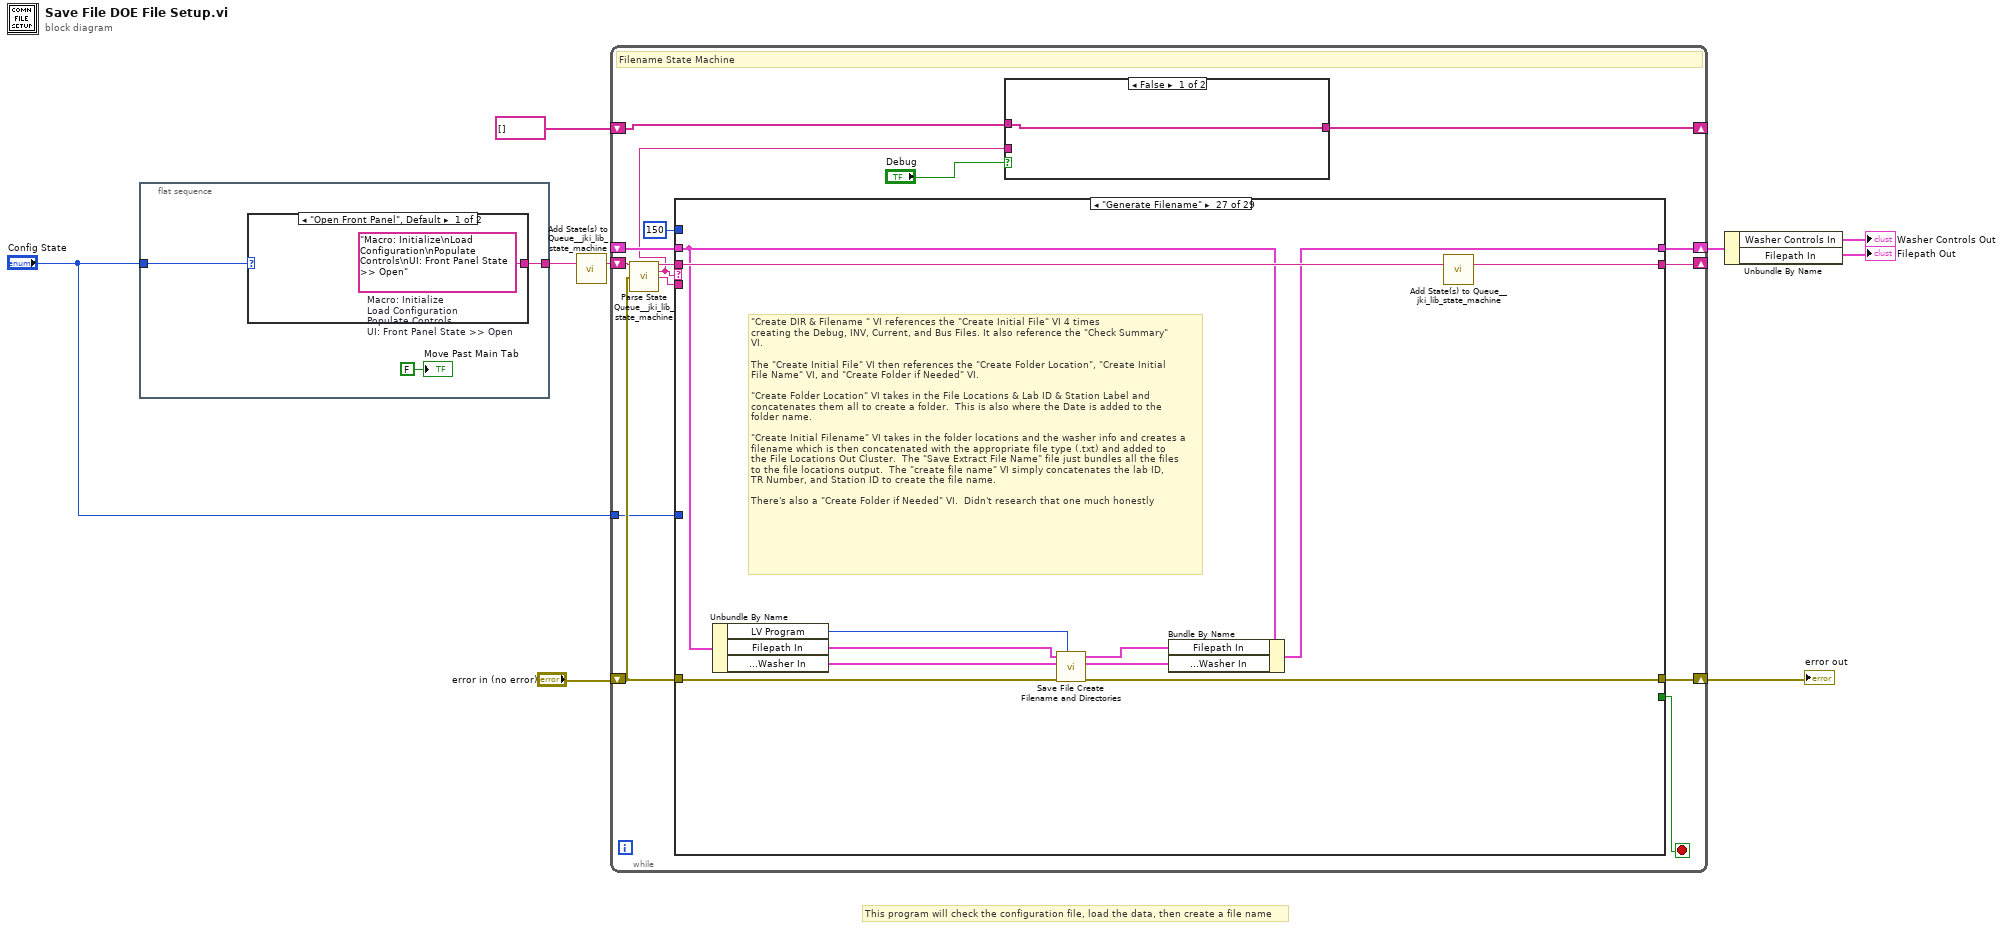
[diagram p0: block diagram]
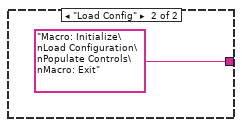
[diagram p2: hidden frame]
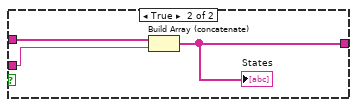
[diagram p3: hidden frame]
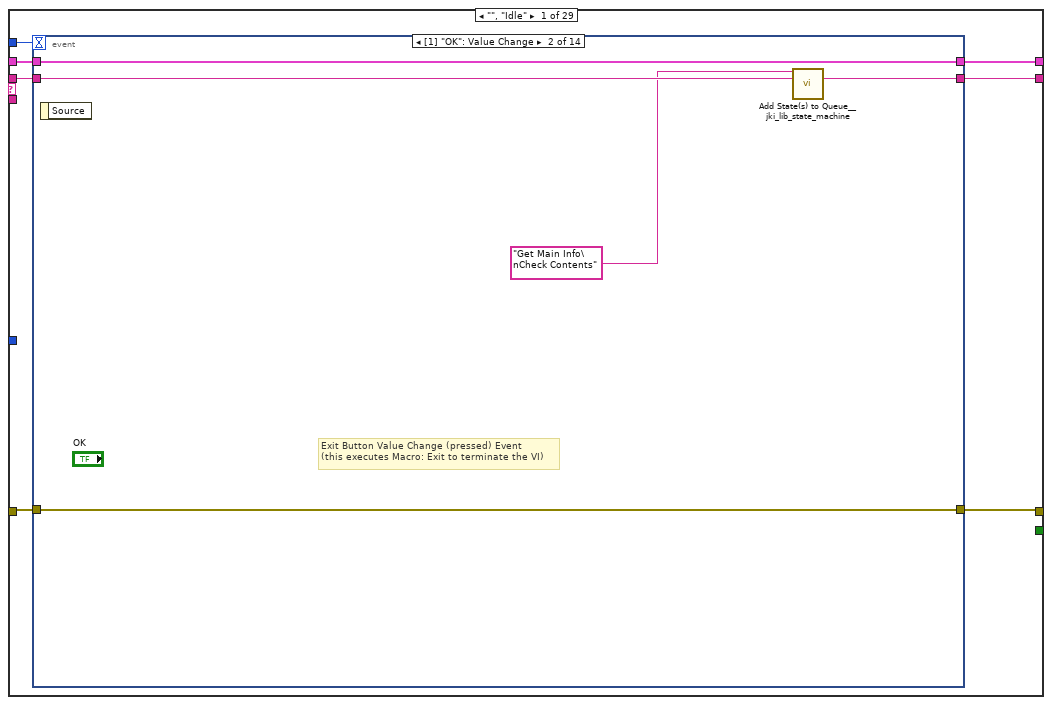
[diagram p4: hidden frame]
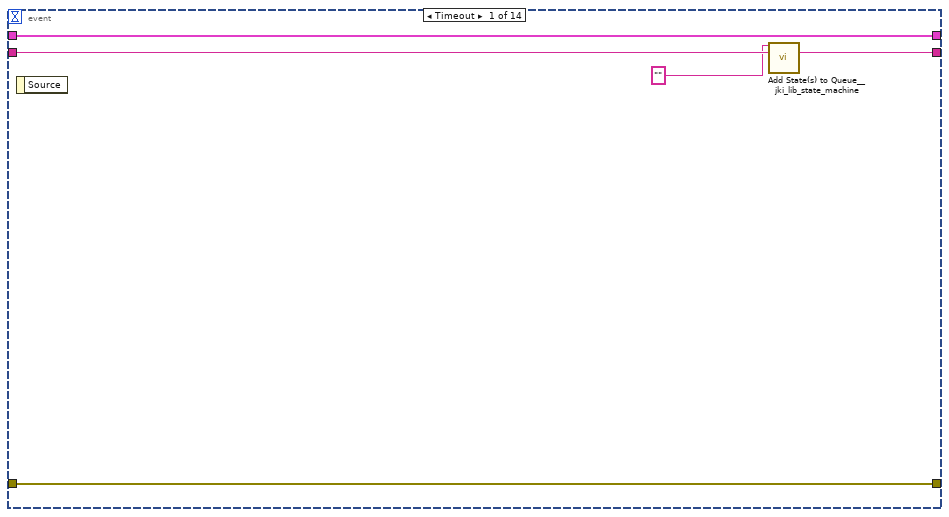
[diagram p5: hidden frame]
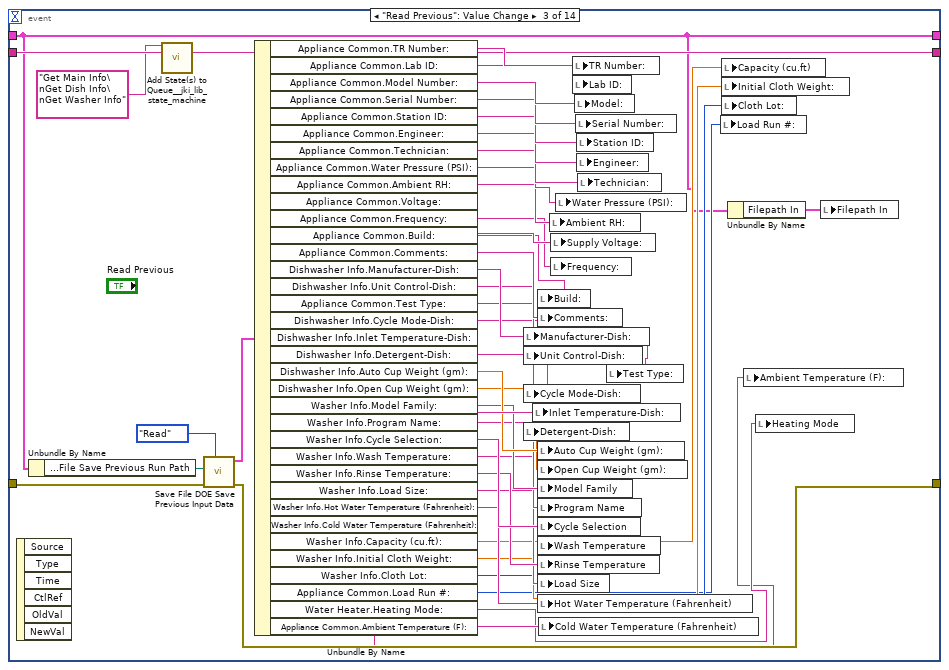
[diagram p6: hidden frame]
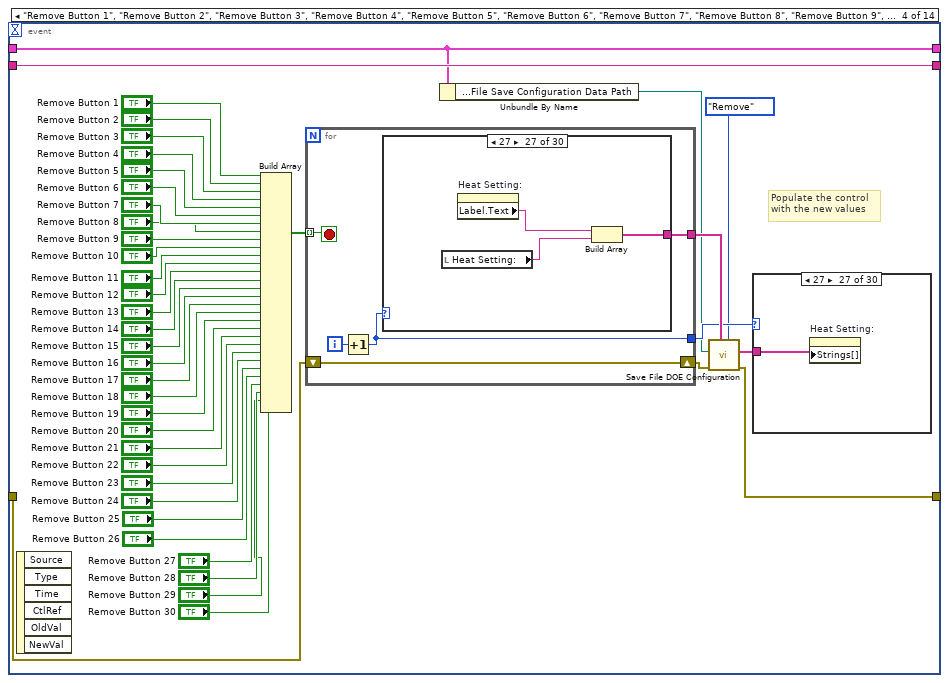
[diagram p7: hidden frame]
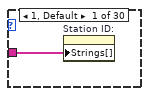
[diagram p8: hidden frame]
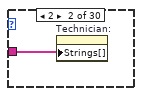
[diagram p9: hidden frame]
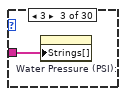
[diagram p10: hidden frame]
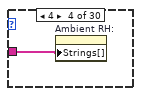
[diagram p11: hidden frame]
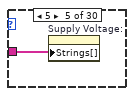
[diagram p12: hidden frame]
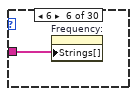
[diagram p13: hidden frame]
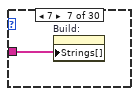
[diagram p14: hidden frame]
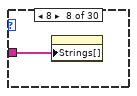
[diagram p15: hidden frame]
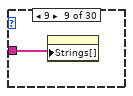
[diagram p16: hidden frame]
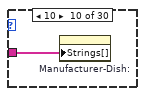
[diagram p17: hidden frame]
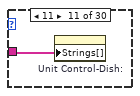
[diagram p18: hidden frame]
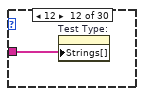
[diagram p19: hidden frame]
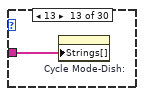
[diagram p20: hidden frame]
diagram:
  # "This program will check the configuration file, load the data, then create a file name"
  n1 = flat-sequence {
    tunnel: [w12] -> w5
    tunnel: "Config State" -> [w10]
    frame #0 {
      n2 = case shown="\"Open Front Panel\", Default" w10 {
        tunnel: [w13 "Macro: Initialize\nLoad Configuration\nPopulate Controls\nMacro: Exit"] -> w12
        frame "Open Front Panel", Default {
          w13 = "Macro: Initialize\nLoad Configuration\nPopulate Controls\nUI: Front Panel State >> Open"  # Macro: Initialize Load Configuration Populate Controls UI: Front Panel State >> Open
        }
        frame "Load Config" {
        }
      }
      "Move Past Main Tab" <- FALSE ("Move Past Main Tab")
    }
  }
  n3 = call <vilib>:"Add State(s) to Queue__jki_lib_state_machine.vi"("State(s) in (\"\")"=w5) -> ("States Out"=w8:string)  [unwired: 14 in]
  n4 = while "Filename State Machine" {
    shift-right: [w23] -> w6
    shift-left: _ -> [w22]
    shift-right: [w26] -> w9
    shift-left: "error in (no error)" -> [w20]
    shift-right: [w25] -> _
    shift-left: w8 -> [w27]
    shift-right: [w18] -> _
    shift-left: string[] [] -> [w19]
    tunnel: "Config State" -> [w15]
    stop <- w24 stop-if-true
    # "Filename State Machine"
    n5 = call <vilib>:"Parse State Queue__jki_lib_state_machine.vi"("State Queue"=w27, "Error In (no error)"=w20) -> ("Remaining States"=w29:string, "Current State"=w17:string, "Arguments"=w28:string)  [unwired: 11 in]
    n6 = case shown="\"Generate Filename\"" w17 {
      selector: w17 -> [_ _ w552 _ _ _ _ _ _ _ _ _ _ _ _ _ _ _ _ _ _ _ _ _ _ _ _ _ _]
      tunnel: w29 -> [w40 w551 w556 w574 w582 w587 w591 w603 w620 w663 w669 w673 w694 w704 w715 w741 w748 w758 w762 w783 w805 w835 w865 w889 w915 w940 w959 w970 w980]
      tunnel: w28 -> [_ _ _ _ _ _ _ _ _ _ _ _ _ w699 w709 _ _ _ _ _ _ _ _ _ _ _ _ _ _]
      tunnel: w22 -> [w38 w548 w554 w566 w577 w585 w588 _ w615 w639 w664 w670 w686 w702 w711 w738 w745 w755 w759 w782 w801 w834 w864 w888 w914 w939 w956 w968 w974]
      tunnel: [w37 w549 w558 w563 errorcluster {"status"=FALSE, "code"=0, "source"=""} ("error out") w584 w589 w600 w618 w661 w665 w671 w682 w700 w712 w739 w746 w756 w760 w785 w803 w837 w867 w891 w917 w942 w949 w960 w971] -> w26
      tunnel: w20 -> [w36 w549 w557 w563 w579 w584 w589 w600 w617 w661 w666 w671 w676 w701 w713 w739 w746 w756 w760 w785 w803 w837 w867 w891 w917 w942 w950 w961 w972]
      tunnel: [w39 w550 w555 w573 w581 w586 w590 w602 w619 w662 w668 w672 w693 w703 w714 w740 w747 w757 w761 w786 w804 w838 w868 w892 w918 w943 w958 w969 w979] -> w25
      tunnel: [_ _ _ _ _ TRUE _ _ _ _ _ _ _ _ _ _ _ _ _ _ _ _ _ _ _ _ _ _ _] -> w24
      tunnel: [w35 w548 w554 w572 w576 w585 w588 w601 w610 w639 w664 w670 w675 w702 w711 w738 w745 w755 w759 w784 w800 w836 w866 w890 w916 w941 w957 w967 w974] -> w23
      tunnel: 150 ("Timeout") -> [w34 _ _ _ _ _ _ _ _ _ _ _ _ _ _ _ _ _ _ _ _ _ _ _ _ _ _ _ _]
      tunnel: w15 -> [_ _ _ _ _ _ _ _ w607 _ _ _ _ _ _ _ _ _ _ _ _ _ _ _ _ _ _ _ _]
      frame "", "Idle" {
        n7 = event shown="[1] \"OK\": Value Change" {
          selector: _ -> [_ _ _ _ _ _ _ _ _ _ _ _ _ _]
          dyn-events: _ -> [_ _ _ _ _ _ _ _ _ _ _ _ _ _]
          timeout: w34 -> [_ _ _ _ _ _ _ _ _ _ _ _ _ _]
          tunnel: w40 -> [w45 w50 w57 w136 w287 w435 w440 w449 w457 w479 w486 w509 w524 w547]
          tunnel: [w44 w49 w56 w136 w287 w434 w440 w449 w457 w479 w486 w509 w525 w546] -> w39
          tunnel: w38 -> [w41 w47 w51 w106 w272 w436 w439 w450 w458 w477 w488 w503 w523 w544]
          tunnel: [w43 w48 w94 w120 w278 w430 w441 w448 w456 w466 w484 w508 w526 w545] -> w37
          tunnel: w36 -> [w43 w48 w95 w113 w280 w430 w442 w448 w456 w460 w485 w506 w526 w545]
          tunnel: [w41 w47 w51 w106 w272 w436 w439 w450 w458 w478 w487 w503 w523 w544] -> w35
          event Timeout {
            n8 = event-data() -> ()  [unwired: 1 in, 1 out]
            n9 = call <vilib>:"Add State(s) to Queue__jki_lib_state_machine.vi"("State(s) in Front (\"\")"="" ("State(s) in Front (\"\")"), "State(s) in (\"\")"=w45) -> ("States Out"=w44:string)  [unwired: 13 in]
          }
          event Value Change {
            # "Exit Button Value Change (pressed) Event\n(this executes Macro: Exit to terminate the VI)"
            n10 = event-data() -> ()  [unwired: 1 in, 1 out]
            n11 = call <vilib>:"Add State(s) to Queue__jki_lib_state_machine.vi"("State(s) in Front (\"\")"="Get Main Info\nCheck Contents", "State(s) in (\"\")"=w50) -> ("States Out"=w49:string)  [unwired: 13 in]
          }
          event "Read Previous": Value Change {
            n12 = event-data() -> ()  [unwired: 1 in, 6 out]
            n13 = Unbundle By Name(w51) -> ("Filepath In.General Setup Paths.File Save Previous Run Path"=w92:path)
            n14 = call <vilib>:"Add State(s) to Queue__jki_lib_state_machine.vi"("State(s) in Front (\"\")"="Get Main Info\nGet Dish Info\nGet Washer Info", "State(s) in (\"\")"=w57) -> ("States Out"=w56:string)  [unwired: 13 in]
            n15 = call "Save File DOE Save Previous Input Data.vi"("State"=enum16{"Write", "Read"}."Read", "error in (no error)"=w95, "Appliance Previous Run Path"=w92) -> ("error out"=w94:errorcluster, "Appliance Details Ouput"=w91:T22)  [unwired: 7 in]
            n16 = Unbundle By Name(w91) -> ("Appliance Common.TR Number:"=w90:string, "Appliance Common.Lab ID:"=w89:string, "Appliance Common.Model Number:"=w88:string, "Appliance Common.Serial Number:"=w87:string, "Appliance Common.Station ID:"=w86:string, "Appliance Common.Engineer:"=w85:string, "Appliance Common.Technician:"=w84:string, "Appliance Common.Water Pressure (PSI):"=w83:string, "Appliance Common.Ambient RH:"=w82:string, "Appliance Common.Voltage:"=w81:string, "Appliance Common.Frequency:"=w80:string, "Appliance Common.Build:"=w79:string, "Appliance Common.Comments:"=w78:string, "Dishwasher Info.Manufacturer-Dish:"=w77:string, "Dishwasher Info.Unit Control-Dish:"=w76:string, "Appliance Common.Test Type:"=w75:string, "Dishwasher Info.Cycle Mode-Dish:"=w74:string, "Dishwasher Info.Inlet Temperature-Dish:"=w73:string, "Dishwasher Info.Detergent-Dish:"=w72:string, "Dishwasher Info.Auto Cup Weight (gm):"=w71:dbl, "Dishwasher Info.Open Cup Weight (gm):"=w70:dbl, "Washer Info.Model Family:"=w69:string, "Washer Info.Program Name:"=w68:string, "Washer Info.Cycle Selection:"=w67:string, "Washer Info.Wash Temperature:"=w66:string, "Washer Info.Rinse Temperature:"=w65:string, "Washer Info.Load Size:"=w64:string, "Washer Info.Hot Water Temperature (Fahrenheit):"=w63:string, "Washer Info.Cold Water Temperature (Fahrenheit):"=w62:string, "Washer Info.Capacity (cu.ft):"=w61:dbl, "Washer Info.Initial Cloth Weight:"=w60:dbl, "Washer Info.Cloth Lot:"=w59:i32, "Appliance Common.Load Run #:"=w58:i32, "Water Heater.Heating Mode:"=w53:string, "Appliance Common.Ambient Temperature (F):"=w52:string)
            n17 = local write "Manufacturer-Dish:"(w77) -> ()
            n18 = local write "Unit Control-Dish:"(w76) -> ()
            n19 = local write "Cycle Mode-Dish:"(w74) -> ()
            n20 = local write "Detergent-Dish:"(w72) -> ()
            n21 = local write "Inlet Temperature-Dish:"(w73) -> ()
            n22 = local write "Build:"(w79) -> ()
            n23 = local write "Comments:"(w78) -> ()
            n24 = local write "Auto Cup Weight (gm):"(w71) -> ()
            n25 = local write "Open Cup Weight (gm):"(w70) -> ()
            n26 = local write "Model Family"(w69) -> ()
            n27 = local write "Program Name"(w68) -> ()
            n28 = local write "Cycle Selection"(w67) -> ()
            n29 = local write "Wash Temperature"(w66) -> ()
            n30 = local write "Rinse Temperature"(w65) -> ()
            n31 = local write "Load Size"(w64) -> ()
            n32 = local write "Hot Water Temperature (Fahrenheit)"(w63) -> ()
            n33 = local write "Cold Water Temperature (Fahrenheit)"(w62) -> ()
            n34 = local write "Ambient RH:"(w82) -> ()
            n35 = local write "Supply Voltage:"(w81) -> ()
            n36 = local write "Frequency:"(w80) -> ()
            n37 = local write "Water Pressure (PSI):"(w83) -> ()
            n38 = local write "TR Number:"(w90) -> ()
            n39 = local write "Lab ID:"(w89) -> ()
            n40 = local write "Model:"(w88) -> ()
            n41 = local write "Serial Number:"(w87) -> ()
            n42 = local write "Station ID:"(w86) -> ()
            n43 = local write "Engineer:"(w85) -> ()
            n44 = local write "Technician:"(w84) -> ()
            n45 = local write "Test Type:"(w75) -> ()
            n46 = local write "Load Run #:"(w58) -> ()
            n47 = local write "Capacity (cu.ft)"(w61) -> ()
            n48 = local write "Initial Cloth Weight:"(w60) -> ()
            n49 = local write "Cloth Lot:"(w59) -> ()
            n50 = Unbundle By Name(w51) -> ("Filepath In"=w54:T10)
            n51 = local write "Ambient Temperature (F):"(w52) -> ()
            n52 = local write "Heating Mode"(w53) -> ()
            n53 = local write "Filepath In"(w54) -> ()
          }
          event "Remove Button 1", "Remove Button 2", "Remove Button 3", "Remove Button 4", "Remove Button 5", "Remove Button 6", "Remove Button 7", "Remove Button 8", "Remove Button 9", "Remove Button 10", "Remove Button 11", "Remove Button 12", "Remove Button 13", "Remove Button 14", "Remove Button 15", "Remove Button 16", "Remove Button 17", "Remove Button 18", "Remove Button 19", "Remove Button 20", "Remove Button 21", "Remove Button 22", "Remove Button 23", "Remove Button 24", "Remove Button 25", "Remove Button 26", "Remove Button 27", "Remove Button 28", "Remove Button 29", "Remove Button 30": Value Change {
            # "Populate the control\nwith the new values"
            n54 = event-data() -> ()  [unwired: 1 in, 6 out]
            n55 = Build Array("Remove Button 1", "Remove Button 2", "Remove Button 3", "Remove Button 4", "Remove Button 5", "Remove Button 6", "Remove Button 7", "Remove Button 8", "Remove Button 9", "Remove Button 10", "Remove Button 11", "Remove Button 12", "Remove Button 13", "Remove Button 14", "Remove Button 15", "Remove Button 16", "Remove Button 17", "Remove Button 18", "Remove Button 19", "Remove Button 20", "Remove Button 21", "Remove Button 22", "Remove Button 23", "Remove Button 24", "Remove Button 25", "Remove Button 26", "Remove Button 27", "Remove Button 28", "Remove Button 29", "Remove Button 30") -> (w117:bool[])
            n56 = for {
              tunnel: w117 -> [w171] mode=indexing
              shift-right: [w169] -> w112
              shift-left: w113 -> [w169]
              tunnel: [w168] -> w109
              tunnel: [w167] -> w111
              i -> [w170]
              stop <- w171 stop-if-true
              n57 = Increment(x=w170) -> (x+1=w168:i32)
              n58 = case shown="27" w168 {
                tunnel: [w172 w175 w178 w181 w184 w187 w191 w193 w196 w199 w202 w205 w208 w211 w214 w217 w220 w223 w226 w229 w233 w235 w238 w241 w244 w247 w251 w253 w256 w259] -> w167
                frame 1, Default {
                  # "Station ID Remove"
                  n59 = property on="Station ID:" class="CmbBox"() -> ("Label.Text"=w173:string)  [unwired: 2 in, 2 out]
                  n60 = local read "Station ID:"() -> (w174:string)
                  n61 = Build Array(w173, w174) -> (w172:string[])
                }
                frame 2 {
                  # "Technician Remove"
                  n62 = property on="Technician:" class="CmbBox"() -> ("Label.Text"=w176:string)  [unwired: 2 in, 2 out]
                  n63 = local read "Technician:"() -> (w177:string)
                  n64 = Build Array(w176, w177) -> (w175:string[])
                }
                frame 3 {
                  # "Water Pressure PSI Remove"
                  n65 = local read "Water Pressure (PSI):"() -> (w179:string)
                  n66 = property on="Water Pressure (PSI):" class="CmbBox"() -> ("Label.Text"=w180:string)  [unwired: 2 in, 2 out]
                  n67 = Build Array(w180, w179) -> (w178:string[])
                }
                frame 4 {
                  # "Ambient RH Remove"
                  n68 = property on="Ambient RH:" class="CmbBox"() -> ("Label.Text"=w183:string)  [unwired: 2 in, 2 out]
                  n69 = local read "Ambient RH:"() -> (w182:string)
                  n70 = Build Array(w183, w182) -> (w181:string[])
                }
                frame 5 {
                  # "Supply Voltage"
                  n71 = property on="Supply Voltage:" class="CmbBox"() -> ("Label.Text"=w185:string)  [unwired: 2 in, 2 out]
                  n72 = local read "Supply Voltage:"() -> (w186:string)
                  n73 = Build Array(w185, w186) -> (w184:string[])
                }
                frame 6 {
                  # "Frequency"
                  n74 = property on="Frequency:" class="CmbBox"() -> ("Label.Text"=w188:string)  [unwired: 2 in, 2 out]
                  n75 = local read "Frequency:"() -> (w189:string)
                  n76 = Build Array(w188, w189) -> (w187:string[])
                }
                frame 7 {
                  # "Build"
                  n77 = property on="Build:" class="CmbBox"() -> ("Label.Text"=w190:string)  [unwired: 2 in, 2 out]
                  n78 = local read "Build:"() -> (w192:string)
                  n79 = Build Array(w190, w192) -> (w191:string[])
                }
                frame 8 {
                  # "Hot Water Temperature (Washer)"
                  n80 = local read "Hot Water Temperature (Fahrenheit)"() -> (w195:string)
                  n81 = property on="Hot Water Temperature (Fahrenheit)" class="CmbBox"() -> ("Label.Text"=w194:string)  [unwired: 2 in, 2 out]
                  n82 = Build Array(w194, w195) -> (w193:string[])
                }
                frame 9 {
                  # "Cold Water Temperature (Washer)"
                  n83 = property on="Cold Water Temperature (Fahrenheit)" class="CmbBox"() -> ("Label.Text"=w197:string)  [unwired: 2 in, 2 out]
                  n84 = local read "Cold Water Temperature (Fahrenheit)"() -> (w198:string)
                  n85 = Build Array(w197, w198) -> (w196:string[])
                }
                frame 10 {
                  # "Manufacturer (Dish)"
                  n86 = local read "Manufacturer-Dish:"() -> (w201:string)
                  n87 = property on="Manufacturer-Dish:" class="CmbBox"() -> ("Label.Text"=w200:string)  [unwired: 2 in, 2 out]
                  n88 = Build Array(w200, w201) -> (w199:string[])
                }
                frame 11 {
                  # "Unit Control (Dish)"
                  n89 = local read "Unit Control-Dish:"() -> (w203:string)
                  n90 = property on="Unit Control-Dish:" class="CmbBox"() -> ("Label.Text"=w204:string)  [unwired: 2 in, 2 out]
                  n91 = Build Array(w204, w203) -> (w202:string[])
                }
                frame 12 {
                  # "Test Type (Dish)"
                  n92 = property on="Test Type:" class="CmbBox"() -> ("Label.Text"=w206:string)  [unwired: 2 in, 2 out]
                  n93 = local read "Test Type:"() -> (w207:string)
                  n94 = Build Array(w206, w207) -> (w205:string[])
                }
                frame 13 {
                  # "Cycle Mode (Dish)"
                  n95 = local read "Cycle Mode-Dish:"() -> (w210:string)
                  n96 = property on="Cycle Mode-Dish:" class="CmbBox"() -> ("Label.Text"=w209:string)  [unwired: 2 in, 2 out]
                  n97 = Build Array(w209, w210) -> (w208:string[])
                }
                frame 14 {
                  # "Inlet Temperature (Dish)"
                  n98 = local read "Inlet Temperature-Dish:"() -> (w213:string)
                  n99 = property on="Inlet Temperature-Dish:" class="CmbBox"() -> ("Label.Text"=w212:string)  [unwired: 2 in, 2 out]
                  n100 = Build Array(w212, w213) -> (w211:string[])
                }
                frame 15 {
                  # "Detergent (Dish)"
                  n101 = local read "Detergent-Dish:"() -> (w216:string)
                  n102 = property on="Detergent-Dish:" class="CmbBox"() -> ("Label.Text"=w215:string)  [unwired: 2 in, 2 out]
                  n103 = Build Array(w215, w216) -> (w214:string[])
                }
                frame 16 {
                  # "TR Number"
                  n104 = property on="TR Number:" class="CmbBox"() -> ("Label.Text"=w218:string)  [unwired: 2 in, 2 out]
                  n105 = local read "TR Number:"() -> (w219:string)
                  n106 = Build Array(w218, w219) -> (w217:string[])
                }
                frame 17 {
                  # "Lab ID Number"
                  n107 = property on="Lab ID:" class="CmbBox"() -> ("Label.Text"=w221:string)  [unwired: 2 in, 2 out]
                  n108 = local read "Lab ID:"() -> (w222:string)
                  n109 = Build Array(w221, w222) -> (w220:string[])
                }
                frame 18 {
                  n110 = property on="Wash Temperature" class="CmbBox"() -> ("Label.Text"=w224:string)  [unwired: 2 in, 2 out]
                  n111 = local read "Wash Temperature"() -> (w225:string)
                  n112 = Build Array(w224, w225) -> (w223:string[])
                }
                frame 19 {
                  n113 = property on="Rinse Temperature" class="CmbBox"() -> ("Label.Text"=w227:string)  [unwired: 2 in, 2 out]
                  n114 = local read "Rinse Temperature"() -> (w228:string)
                  n115 = Build Array(w227, w228) -> (w226:string[])
                }
                frame 20 {
                  n116 = property on="Load Size" class="CmbBox"() -> ("Label.Text"=w230:string)  [unwired: 2 in, 2 out]
                  n117 = local read "Load Size"() -> (w231:string)
                  n118 = Build Array(w230, w231) -> (w229:string[])
                }
                frame 21 {
                  n119 = property on="Cycle Selection" class="CmbBox"() -> ("Label.Text"=w232:string)  [unwired: 2 in, 2 out]
                  n120 = local read "Cycle Selection"() -> (w234:string)
                  n121 = Build Array(w232, w234) -> (w233:string[])
                }
                frame 22 {
                  n122 = property on="Heating Mode" class="CmbBox (strict)"() -> ("Label.Text"=w236:string)  [unwired: 2 in, 2 out]
                  n123 = local read "Heating Mode"() -> (w237:T4)
                  n124 = Build Array(w236, w237) -> (w235:T4[])
                }
                frame 23 {
                  n125 = local read "Ambient Temperature (F):"() -> (w239:string)
                  n126 = property on="Ambient Temperature (F):" class="CmbBox"() -> ("Label.Text"=w240:string)  [unwired: 2 in, 2 out]
                  n127 = Build Array(w240, w239) -> (w238:string[])
                }
                frame 24 {
                  n128 = local read "Dryer Type:"() -> (w242:string)
                  n129 = property on="Dryer Type:" class="CmbBox"() -> ("Label.Text"=w243:string)  [unwired: 2 in, 2 out]
                  n130 = Build Array(w243, w242) -> (w241:string[])
                }
                frame 25 {
                  n131 = local read "Exhaust:"() -> (w245:string)
                  n132 = property on="Exhaust:" class="CmbBox"() -> ("Label.Text"=w246:string)  [unwired: 2 in, 2 out]
                  n133 = Build Array(w246, w245) -> (w244:string[])
                }
                frame 26 {
                  n134 = local read "Drying Cycle:"() -> (w248:string)
                  n135 = property on="Drying Cycle:" class="CmbBox"() -> ("Label.Text"=w249:string)  [unwired: 2 in, 2 out]
                  n136 = Build Array(w249, w248) -> (w247:string[])
                }
                frame 27 {
                  n137 = local read "Heat Setting:"() -> (w250:string)
                  n138 = property on="Heat Setting:" class="CmbBox"() -> ("Label.Text"=w252:string)  [unwired: 2 in, 2 out]
                  n139 = Build Array(w252, w250) -> (w251:string[])
                }
                frame 28 {
                  n140 = local read "Dryness Setting:"() -> (w254:string)
                  n141 = property on="Dryness Setting:" class="CmbBox"() -> ("Label.Text"=w255:string)  [unwired: 2 in, 2 out]
                  n142 = Build Array(w255, w254) -> (w253:string[])
                }
                frame 29 {
                  n143 = local read "Nominal Load Weight (lbs):"() -> (w257:string)
                  n144 = property on="Nominal Load Weight (lbs):" class="CmbBox"() -> ("Label.Text"=w258:string)  [unwired: 2 in, 2 out]
                  n145 = Build Array(w258, w257) -> (w256:string[])
                }
                frame 30 {
                  n146 = local read "Load Type:"() -> (w260:string)
                  n147 = property on="Load Type:" class="CmbBox"() -> ("Label.Text"=w261:string)  [unwired: 2 in, 2 out]
                  n148 = Build Array(w261, w260) -> (w259:string[])
                }
              }
            }
            n149 = Unbundle By Name(w106) -> ("Filepath In.General Setup Paths.File Save Configuration Data Path"=w105:path)
            n150 = call "Save File DOE Configuration.vi"("Add/Remove Enum"=T27."Remove", "Latest String Search"=w111, "error in (no error)"=w112, "File Save Configuration Data Path"=w105) -> ("error out"=w120:errorcluster, "Updated List"=w108:string[])  [unwired: 5 in, 1 out]
            n151 = case shown="27" w109 {
              tunnel: w108 -> [w137 w138 w139 w140 w141 w142 w143 w144 w145 w146 w147 w148 w149 w150 w151 w152 w153 w154 w155 w156 w157 w158 w159 w160 w161 w162 w163 w164 w165 w166]
              frame 1, Default {
                n152 = property on="Station ID:" class="CmbBox"("Strings[]"=w137) -> ()  [unwired: 2 in, 2 out]
              }
              frame 2 {
                n153 = property on="Technician:" class="CmbBox"("Strings[]"=w138) -> ()  [unwired: 2 in, 2 out]
              }
              frame 3 {
                n154 = property on="Water Pressure (PSI):" class="CmbBox"("Strings[]"=w139) -> ()  [unwired: 2 in, 2 out]
              }
              frame 4 {
                n155 = property on="Ambient RH:" class="CmbBox"("Strings[]"=w140) -> ()  [unwired: 2 in, 2 out]
              }
              frame 5 {
                n156 = property on="Supply Voltage:" class="CmbBox"("Strings[]"=w141) -> ()  [unwired: 2 in, 2 out]
              }
              frame 6 {
                n157 = property on="Frequency:" class="CmbBox"("Strings[]"=w142) -> ()  [unwired: 2 in, 2 out]
              }
              frame 7 {
                n158 = property on="Build:" class="CmbBox"("Strings[]"=w143) -> ()  [unwired: 2 in, 2 out]
              }
              frame 8 {
                n159 = property on="Hot Water Temperature (Fahrenheit)" class="CmbBox"("Strings[]"=w144) -> ()  [unwired: 2 in, 2 out]
              }
              frame 9 {
                n160 = property on="Cold Water Temperature (Fahrenheit)" class="CmbBox"("Strings[]"=w145) -> ()  [unwired: 2 in, 2 out]
              }
              frame 10 {
                n161 = property on="Manufacturer-Dish:" class="CmbBox"("Strings[]"=w146) -> ()  [unwired: 2 in, 2 out]
              }
              frame 11 {
                n162 = property on="Unit Control-Dish:" class="CmbBox"("Strings[]"=w147) -> ()  [unwired: 2 in, 2 out]
              }
              frame 12 {
                n163 = property on="Test Type:" class="CmbBox"("Strings[]"=w148) -> ()  [unwired: 2 in, 2 out]
              }
              frame 13 {
                n164 = property on="Cycle Mode-Dish:" class="CmbBox"("Strings[]"=w149) -> ()  [unwired: 2 in, 2 out]
              }
              frame 14 {
                n165 = property on="Inlet Temperature-Dish:" class="CmbBox"("Strings[]"=w150) -> ()  [unwired: 2 in, 2 out]
              }
              frame 15 {
                n166 = property on="Detergent-Dish:" class="CmbBox"("Strings[]"=w151) -> ()  [unwired: 2 in, 2 out]
              }
              frame 16 {
                n167 = property on="TR Number:" class="CmbBox"("Strings[]"=w152) -> ()  [unwired: 2 in, 2 out]
              }
              frame 17 {
                n168 = property on="Lab ID:" class="CmbBox"("Strings[]"=w153) -> ()  [unwired: 2 in, 2 out]
              }
              frame 18 {
                n169 = property on="Wash Temperature" class="CmbBox"("Strings[]"=w154) -> ()  [unwired: 2 in, 2 out]
              }
              frame 19 {
                n170 = property on="Rinse Temperature" class="CmbBox"("Strings[]"=w155) -> ()  [unwired: 2 in, 2 out]
              }
              frame 20 {
                n171 = property on="Load Size" class="CmbBox"("Strings[]"=w156) -> ()  [unwired: 2 in, 2 out]
              }
              frame 21 {
                n172 = property on="Cycle Selection" class="CmbBox"("Strings[]"=w157) -> ()  [unwired: 2 in, 2 out]
              }
              frame 22 {
                n173 = property on="Heating Mode" class="CmbBox (strict)"("Strings[]"=w158) -> ()  [unwired: 2 in, 2 out]
              }
              frame 23 {
                n174 = property on="Ambient Temperature (F):" class="CmbBox"("Strings[]"=w159) -> ()  [unwired: 2 in, 2 out]
              }
              frame 24 {
                n175 = property on="Dryer Type:" class="CmbBox"("Strings[]"=w160) -> ()  [unwired: 2 in, 2 out]
              }
              frame 25 {
                n176 = property on="Exhaust:" class="CmbBox"("Strings[]"=w161) -> ()  [unwired: 2 in, 2 out]
              }
              frame 26 {
                n177 = property on="Drying Cycle:" class="CmbBox"("Strings[]"=w162) -> ()  [unwired: 2 in, 2 out]
              }
              frame 27 {
                n178 = property on="Heat Setting:" class="CmbBox"("Strings[]"=w163) -> ()  [unwired: 2 in, 2 out]
              }
              frame 28 {
                n179 = property on="Dryness Setting:" class="CmbBox"("Strings[]"=w164) -> ()  [unwired: 2 in, 2 out]
              }
              frame 29 {
                n180 = property on="Nominal Load Weight (lbs):" class="CmbBox"("Strings[]"=w165) -> ()  [unwired: 2 in, 2 out]
              }
              frame 30 {
                n181 = property on="Load Type:" class="CmbBox"("Strings[]"=w166) -> ()  [unwired: 2 in, 2 out]
              }
            }
          }
          event "Add Button 1", "Add Button 2", "Add Button 3", "Add Button 4", "Add Button 5", "Add Button 6", "Add Button 7", "Add Button 8", "Add Button 9", "Add Button 10", "Add Button 11", "Add Button 12", "Add Button 13", "Add Button 14", "Add Button 15", "Add Button 16", "Add Button 17", "Add Button 18", "Add Button 19", "Add Button 20", "Add Button 21", "Add Button 22", "Add Button 23", "Add Button 24", "Add Button 25", "Add Button 26", "Add Button 27", "Add Button 28", "Add Button 29", "Add Button 30": Value Change {
            n182 = event-data() -> ()  [unwired: 1 in, 6 out]
            n183 = Build Array("Add Button 1", "Add Button 2", "Add Button 3", "Add Button 4", "Add Button 5", "Add Button 6", "Add Button 7", "Add Button 8", "Add Button 9", "Add Button 10", "Add Button 11", "Add Button 12", "Add Button 13", "Add Button 14", "Add Button 15", "Add Button 16", "Add Button 17", "Add Button 18", "Add Button 19", "Add Button 20", "Add Button 21", "Add Button 22", "Add Button 23", "Add Button 24", "Add Button 25", "Add Button 26", "Add Button 27", "Add Button 28", "Add Button 29", "Add Button 30") -> (w281:bool[])
            n184 = for {
              tunnel: w281 -> [w337] mode=indexing
              shift-right: [w335] -> w279
              shift-left: w280 -> [w335]
              tunnel: [w333] -> w274
              tunnel: [w334] -> w277
              i -> [w336]
              stop <- w337 stop-if-true
              n185 = Increment(x=w336) -> (x+1=w333:i32)
              n186 = case shown="23" w333 {
                tunnel: [w338 w341 w344 w347 w350 w353 w357 w359 w362 w365 w368 w371 w374 w377 w380 w383 w386 w389 w392 w395 w399 w401 w404 w407 w410 w413 w418 w421 w423 w426] -> w334
                frame 1, Default {
                  # "Station ID Remove"
                  n187 = property on="Station ID:" class="CmbBox"() -> ("Label.Text"=w339:string)  [unwired: 2 in, 2 out]
                  n188 = local read "Station ID:"() -> (w340:string)
                  n189 = Build Array(w339, w340) -> (w338:string[])
                }
                frame 2 {
                  # "Technician Remove"
                  n190 = property on="Technician:" class="CmbBox"() -> ("Label.Text"=w342:string)  [unwired: 2 in, 2 out]
                  n191 = local read "Technician:"() -> (w343:string)
                  n192 = Build Array(w342, w343) -> (w341:string[])
                }
                frame 3 {
                  # "Water Pressure PSI Remove"
                  n193 = local read "Water Pressure (PSI):"() -> (w345:string)
                  n194 = property on="Water Pressure (PSI):" class="CmbBox"() -> ("Label.Text"=w346:string)  [unwired: 2 in, 2 out]
                  n195 = Build Array(w346, w345) -> (w344:string[])
                }
                frame 4 {
                  # "Ambient RH Remove"
                  n196 = property on="Ambient RH:" class="CmbBox"() -> ("Label.Text"=w349:string)  [unwired: 2 in, 2 out]
                  n197 = local read "Ambient RH:"() -> (w348:string)
                  n198 = Build Array(w349, w348) -> (w347:string[])
                }
                frame 5 {
                  # "Supply Voltage"
                  n199 = property on="Supply Voltage:" class="CmbBox"() -> ("Label.Text"=w351:string)  [unwired: 2 in, 2 out]
                  n200 = local read "Supply Voltage:"() -> (w352:string)
                  n201 = Build Array(w351, w352) -> (w350:string[])
                }
                frame 6 {
                  # "Frequency"
                  n202 = property on="Frequency:" class="CmbBox"() -> ("Label.Text"=w354:string)  [unwired: 2 in, 2 out]
                  n203 = local read "Frequency:"() -> (w355:string)
                  n204 = Build Array(w354, w355) -> (w353:string[])
                }
                frame 7 {
                  # "Build"
                  n205 = property on="Build:" class="CmbBox"() -> ("Label.Text"=w356:string)  [unwired: 2 in, 2 out]
                  n206 = local read "Build:"() -> (w358:string)
                  n207 = Build Array(w356, w358) -> (w357:string[])
                }
                frame 8 {
                  # "Hot Water Temperature (Washer)"
                  n208 = local read "Hot Water Temperature (Fahrenheit)"() -> (w361:string)
                  n209 = property on="Hot Water Temperature (Fahrenheit)" class="CmbBox"() -> ("Label.Text"=w360:string)  [unwired: 2 in, 2 out]
                  n210 = Build Array(w360, w361) -> (w359:string[])
                }
                frame 9 {
                  # "Cold Water Temperature (Washer)"
                  n211 = property on="Cold Water Temperature (Fahrenheit)" class="CmbBox"() -> ("Label.Text"=w363:string)  [unwired: 2 in, 2 out]
                  n212 = local read "Cold Water Temperature (Fahrenheit)"() -> (w364:string)
                  n213 = Build Array(w363, w364) -> (w362:string[])
                }
                frame 10 {
                  # "Manufacturer (Dish)"
                  n214 = local read "Manufacturer-Dish:"() -> (w367:string)
                  n215 = property on="Manufacturer-Dish:" class="CmbBox"() -> ("Label.Text"=w366:string)  [unwired: 2 in, 2 out]
                  n216 = Build Array(w366, w367) -> (w365:string[])
                }
                frame 11 {
                  # "Unit Control (Dish)"
                  n217 = local read "Unit Control-Dish:"() -> (w369:string)
                  n218 = property on="Unit Control-Dish:" class="CmbBox"() -> ("Label.Text"=w370:string)  [unwired: 2 in, 2 out]
                  n219 = Build Array(w370, w369) -> (w368:string[])
                }
                frame 12 {
                  # "Test Type"
                  n220 = property on="Test Type:" class="CmbBox"() -> ("Label.Text"=w372:string)  [unwired: 2 in, 2 out]
                  n221 = local read "Test Type:"() -> (w373:string)
                  n222 = Build Array(w372, w373) -> (w371:string[])
                }
                frame 13 {
                  # "Cycle Mode (Dish)"
                  n223 = local read "Cycle Mode-Dish:"() -> (w376:string)
                  n224 = property on="Cycle Mode-Dish:" class="CmbBox"() -> ("Label.Text"=w375:string)  [unwired: 2 in, 2 out]
                  n225 = Build Array(w375, w376) -> (w374:string[])
                }
                frame 14 {
                  # "Inlet Temperature (Dish)"
                  n226 = local read "Inlet Temperature-Dish:"() -> (w379:string)
                  n227 = property on="Inlet Temperature-Dish:" class="CmbBox"() -> ("Label.Text"=w378:string)  [unwired: 2 in, 2 out]
                  n228 = Build Array(w378, w379) -> (w377:string[])
                }
                frame 15 {
                  # "Detergent (Dish)"
                  n229 = local read "Detergent-Dish:"() -> (w382:string)
                  n230 = property on="Detergent-Dish:" class="CmbBox"() -> ("Label.Text"=w381:string)  [unwired: 2 in, 2 out]
                  n231 = Build Array(w381, w382) -> (w380:string[])
                }
                frame 16 {
                  # "TR Number"
                  n232 = property on="TR Number:" class="CmbBox"() -> ("Label.Text"=w384:string)  [unwired: 2 in, 2 out]
                  n233 = local read "TR Number:"() -> (w385:string)
                  n234 = Build Array(w384, w385) -> (w383:string[])
                }
                frame 17 {
                  # "Lab ID Number"
                  n235 = property on="Lab ID:" class="CmbBox"() -> ("Label.Text"=w387:string)  [unwired: 2 in, 2 out]
                  n236 = local read "Lab ID:"() -> (w388:string)
                  n237 = Build Array(w387, w388) -> (w386:string[])
                }
                frame 18 {
                  n238 = property on="Wash Temperature" class="CmbBox"() -> ("Label.Text"=w390:string)  [unwired: 2 in, 2 out]
                  n239 = local read "Wash Temperature"() -> (w391:string)
                  n240 = Build Array(w390, w391) -> (w389:string[])
                }
                frame 19 {
                  n241 = property on="Rinse Temperature" class="CmbBox"() -> ("Label.Text"=w393:string)  [unwired: 2 in, 2 out]
                  n242 = local read "Rinse Temperature"() -> (w394:string)
                  n243 = Build Array(w393, w394) -> (w392:string[])
                }
                frame 20 {
                  n244 = property on="Load Size" class="CmbBox"() -> ("Label.Text"=w396:string)  [unwired: 2 in, 2 out]
                  n245 = local read "Load Size"() -> (w397:string)
                  n246 = Build Array(w396, w397) -> (w395:string[])
                }
                frame 21 {
                  n247 = property on="Cycle Selection" class="CmbBox"() -> ("Label.Text"=w398:string)  [unwired: 2 in, 2 out]
                  n248 = local read "Cycle Selection"() -> (w400:string)
                  n249 = Build Array(w398, w400) -> (w399:string[])
                }
                frame 22 {
                  n250 = property on="Heating Mode" class="CmbBox (strict)"() -> ("Label.Text"=w402:string)  [unwired: 2 in, 2 out]
                  n251 = local read "Heating Mode"() -> (w403:T4)
                  n252 = Build Array(w402, w403) -> (w401:T4[])
                }
                frame 23 {
                  n253 = local read "Ambient Temperature (F):"() -> (w405:string)
                  n254 = property on="Ambient Temperature (F):" class="CmbBox"() -> ("Label.Text"=w406:string)  [unwired: 2 in, 2 out]
                  n255 = Build Array(w406, w405) -> (w404:string[])
                }
                frame 24 {
                  n256 = local read "Dryer Type:"() -> (w408:string)
                  n257 = property on="Dryer Type:" class="CmbBox"() -> ("Label.Text"=w409:string)  [unwired: 2 in, 2 out]
                  n258 = Build Array(w409, w408) -> (w407:string[])
                }
                frame 25 {
                  n259 = local read "Exhaust:"() -> (w411:string)
                  n260 = property on="Exhaust:" class="CmbBox"() -> ("Label.Text"=w412:string)  [unwired: 2 in, 2 out]
                  n261 = Build Array(w412, w411) -> (w410:string[])
                }
                frame 26 {
                  n262 = local read "Drying Cycle:"() -> (w414:string)
                  n263 = property on="Drying Cycle:" class="CmbBox"() -> ("Label.Text"=w415:string)  [unwired: 2 in, 2 out]
                  n264 = Build Array(w415, w414) -> (w413:string[])
                }
                frame 27 {
                  n265 = local read "Heat Setting:"() -> (w416:string)
                  n266 = property on="Heat Setting:" class="CmbBox"() -> ("Label.Text"=w417:string)  [unwired: 2 in, 2 out]
                  n267 = Build Array(w417, w416) -> (w418:string[])
                }
                frame 28 {
                  n268 = local read "Dryness Setting:"() -> (w419:string)
                  n269 = property on="Dryness Setting:" class="CmbBox"() -> ("Label.Text"=w420:string)  [unwired: 2 in, 2 out]
                  n270 = Build Array(w420, w419) -> (w421:string[])
                }
                frame 29 {
                  n271 = local read "Nominal Load Weight (lbs):"() -> (w422:string)
                  n272 = property on="Nominal Load Weight (lbs):" class="CmbBox"() -> ("Label.Text"=w424:string)  [unwired: 2 in, 2 out]
                  n273 = Build Array(w424, w422) -> (w423:string[])
                }
                frame 30 {
                  n274 = local read "Load Type:"() -> (w425:string)
                  n275 = property on="Load Type:" class="CmbBox"() -> ("Label.Text"=w427:string)  [unwired: 2 in, 2 out]
                  n276 = Build Array(w427, w425) -> (w426:string[])
                }
              }
            }
            n277 = Unbundle By Name(w272) -> ("Filepath In.General Setup Paths.File Save Configuration Data Path"=w271:path)
            n278 = call "Save File DOE Configuration.vi"("Add/Remove Enum"=T27."Add", "Latest String Search"=w277, "error in (no error)"=w279, "File Save Configuration Data Path"=w271, "Button Number"=w274) -> ("error out"=w278:errorcluster, "Updated List"=w275:string[])  [unwired: 4 in, 1 out]
            n279 = case shown="23" w274 {
              tunnel: w275 -> [w303 w304 w305 w306 w307 w308 w309 w310 w311 w312 w313 w314 w315 w316 w317 w318 w319 w320 w321 w322 w323 w324 w325 w326 w327 w328 w329 w330 w331 w332]
              frame 1, Default {
                n280 = property on="Station ID:" class="CmbBox"("Strings[]"=w303) -> ()  [unwired: 2 in, 2 out]
              }
              frame 2 {
                n281 = property on="Technician:" class="CmbBox"("Strings[]"=w304) -> ()  [unwired: 2 in, 2 out]
              }
              frame 3 {
                n282 = property on="Water Pressure (PSI):" class="CmbBox"("Strings[]"=w305) -> ()  [unwired: 2 in, 2 out]
              }
              frame 4 {
                n283 = property on="Ambient RH:" class="CmbBox"("Strings[]"=w306) -> ()  [unwired: 2 in, 2 out]
              }
              frame 5 {
                n284 = property on="Supply Voltage:" class="CmbBox"("Strings[]"=w307) -> ()  [unwired: 2 in, 2 out]
              }
              frame 6 {
                n285 = property on="Frequency:" class="CmbBox"("Strings[]"=w308) -> ()  [unwired: 2 in, 2 out]
              }
              frame 7 {
                n286 = property on="Build:" class="CmbBox"("Strings[]"=w309) -> ()  [unwired: 2 in, 2 out]
              }
              frame 8 {
                n287 = property on="Hot Water Temperature (Fahrenheit)" class="CmbBox"("Strings[]"=w310) -> ()  [unwired: 2 in, 2 out]
              }
              frame 9 {
                n288 = property on="Cold Water Temperature (Fahrenheit)" class="CmbBox"("Strings[]"=w311) -> ()  [unwired: 2 in, 2 out]
              }
              frame 10 {
                n289 = property on="Manufacturer-Dish:" class="CmbBox"("Strings[]"=w312) -> ()  [unwired: 2 in, 2 out]
              }
              frame 11 {
                n290 = property on="Unit Control-Dish:" class="CmbBox"("Strings[]"=w313) -> ()  [unwired: 2 in, 2 out]
              }
              frame 12 {
                n291 = property on="Test Type:" class="CmbBox"("Strings[]"=w314) -> ()  [unwired: 2 in, 2 out]
              }
              frame 13 {
                n292 = property on="Cycle Mode-Dish:" class="CmbBox"("Strings[]"=w315) -> ()  [unwired: 2 in, 2 out]
              }
              frame 14 {
                n293 = property on="Inlet Temperature-Dish:" class="CmbBox"("Strings[]"=w316) -> ()  [unwired: 2 in, 2 out]
              }
              frame 15 {
                n294 = property on="Detergent-Dish:" class="CmbBox"("Strings[]"=w317) -> ()  [unwired: 2 in, 2 out]
              }
              frame 16 {
                n295 = property on="TR Number:" class="CmbBox"("Strings[]"=w318) -> ()  [unwired: 2 in, 2 out]
              }
              frame 17 {
                n296 = property on="Lab ID:" class="CmbBox"("Strings[]"=w319) -> ()  [unwired: 2 in, 2 out]
              }
              frame 18 {
                n297 = property on="Wash Temperature" class="CmbBox"("Strings[]"=w320) -> ()  [unwired: 2 in, 2 out]
              }
              frame 19 {
                n298 = property on="Rinse Temperature" class="CmbBox"("Strings[]"=w321) -> ()  [unwired: 2 in, 2 out]
              }
              frame 20 {
                n299 = property on="Load Size" class="CmbBox"("Strings[]"=w322) -> ()  [unwired: 2 in, 2 out]
              }
              frame 21 {
                n300 = property on="Cycle Selection" class="CmbBox"("Strings[]"=w323) -> ()  [unwired: 2 in, 2 out]
              }
              frame 22 {
                n301 = property on="Heating Mode" class="CmbBox (strict)"("Strings[]"=w324) -> ()  [unwired: 2 in, 2 out]
              }
              frame 23 {
                n302 = property on="Ambient Temperature (F):" class="CmbBox"("Strings[]"=w325) -> ()  [unwired: 2 in, 2 out]
              }
              frame 24 {
                n303 = property on="Dryer Type:" class="CmbBox"("Strings[]"=w326) -> ()  [unwired: 2 in, 2 out]
              }
              frame 25 {
                n304 = property on="Exhaust:" class="CmbBox"("Strings[]"=w327) -> ()  [unwired: 2 in, 2 out]
              }
              frame 26 {
                n305 = property on="Drying Cycle:" class="CmbBox"("Strings[]"=w328) -> ()  [unwired: 2 in, 2 out]
              }
              frame 27 {
                n306 = property on="Heat Setting:" class="CmbBox"("Strings[]"=w329) -> ()  [unwired: 2 in, 2 out]
              }
              frame 28 {
                n307 = property on="Dryness Setting:" class="CmbBox"("Strings[]"=w330) -> ()  [unwired: 2 in, 2 out]
              }
              frame 29 {
                n308 = property on="Nominal Load Weight (lbs):" class="CmbBox"("Strings[]"=w331) -> ()  [unwired: 2 in, 2 out]
              }
              frame 30 {
                n309 = property on="Load Type:" class="CmbBox"("Strings[]"=w332) -> ()  [unwired: 2 in, 2 out]
              }
            }
          }
          event "Initialize Default": Value Change {
            # "Read the default config file"
            # "Write default values to the main Config File"
            # "Send it back to load configuration to \npopulate the controls"
            n310 = event-data() -> ()  [unwired: 1 in, 6 out]
            n311 = Unbundle By Name(w436) -> ("Filepath In.General Setup Paths.General Startup Config Path"=w431:path)
            n312 = call "Save File DOE Reinitialize Drop Downs to Default.vi"("Save Default"=enum16{"Standard", "Save To Default"}."Standard") -> ("Default Data"=w428:string[][])  [unwired: 9 in, 1 out]
            n313 = call-poly <vilib>:"Write To Spreadsheet File.vi"("delimiter (\\t)"="," ("delimiter (\\t)"), "2D data"=w428, "file path (dialog if empty)"=w431) -> ()  [unwired: 5 in, 1 out]
            n314 = call <vilib>:"Add State(s) to Queue__jki_lib_state_machine.vi"("State(s) in Front (\"\")"="Load Configuration" ("State(s) in Front (\"\")"), "State(s) in (\"\")"=w435) -> ("States Out"=w434:string)  [unwired: 13 in]
          }
          event "Save As Default": Value Change {
            # "Read the default config file"
            n315 = event-data() -> ()  [unwired: 1 in, 6 out]
            n316 = Unbundle By Name(w439) -> ("Filepath In.General Setup Paths.General Startup Config Path"=w438:path)
            n317 = call "Save File DOE Reinitialize Drop Downs to Default.vi"("Save Default"=enum16{"Standard", "Save To Default"}."Save To Default", "error in (no error)"=w442, "Standard Path"=w438) -> ("error out"=w441:errorcluster)  [unwired: 7 in, 1 out]
          }
          event "Get Model Number": Value Change {
            w444 = GEA2_Commands."RQST_MODEL_NUMBER" ("GEA2 Commands and Requests")
            n318 = event-data() -> ()  [unwired: 1 in, 6 out]
            n319 = call "HEWH_DSM_CMD.vi"("GEA2 Commands and Requests"=w444) -> ("Input Data"=w446:T31)  [unwired: 8 in, 1 out]
            n320 = call "GEA2 Send and Receive Message.vi"("Input Data"=w446) -> ("Converted Data Out"=w447:T32)  [unwired: 9 in, 5 out]
            n321 = call "GEA2 Message Decoder.vi"("GEA2 Commands and Requests"=w444, "Coverted Data Out"=w447) -> ("GEA Information Out"=w445:T33)  [unwired: 9 in]
            n322 = Unbundle By Name(w445) -> ("Water Heater GEA2 Data.Extra Data.MODEL NUMBER"=w443:string)
            n323 = local write "Model:"(w443) -> ()
          }
          event "Get Serial Number": Value Change {
            w452 = GEA2_Commands."RQST_SERIAL_NUMBER" ("GEA2 Commands and Requests")
            n324 = event-data() -> ()  [unwired: 1 in, 6 out]
            n325 = call "HEWH_DSM_CMD.vi"("GEA2 Commands and Requests"=w452) -> ("Input Data"=w454:T31)  [unwired: 8 in, 1 out]
            n326 = call "GEA2 Send and Receive Message.vi"("Input Data"=w454) -> ("Converted Data Out"=w455:T32)  [unwired: 9 in, 5 out]
            n327 = call "GEA2 Message Decoder.vi"("GEA2 Commands and Requests"=w452, "Coverted Data Out"=w455) -> ("GEA Information Out"=w453:T33)  [unwired: 9 in]
            n328 = Unbundle By Name(w453) -> ("Water Heater GEA2 Data.Extra Data.SERIAL_NUMBER"=w451:string)
            n329 = local write "Serial Number:"(w451) -> ()
          }
          event "Get Data": Value Change {
            n330 = event-data() -> ()  [unwired: 1 in, 6 out]
            n331 = Unbundle By Name(w477) -> ("Washer Controls In.Initialize.Washer In.Appliance Details.Dryer.Dryer Initial IMC Data"=w476:T25, "Washer Controls In.Test Fixture Hardware.Weight Scale.Com Options.Setra Scale VISA"=w463:refnum<visa-resource-name>)
            n332 = call "ICS425.vi"("VISA resource name"=w463, "Runtime Gather?"=TRUE, "Error In"=w460) -> ("Weight Output"=w461:dbl, "Error Out"=w459:errorcluster)  [unwired: 10 in, 1 out]
            n333 = disable-structure shown="Disabled" {
              frame Disabled {
                n334 = call "Setra Main.vi"() -> ()  [unwired: 13 in, 3 out]
              }
              frame Enabled {
              }
            }
            n335 = property on="Measured Weight (lbf)" class="DigNum (strict)"("Value"=w461) -> ()  [unwired: 2 in, 2 out]
            n336 = Bundle By Name(cluster=w476, "Bone Dry Wt(lbs)"="Bone Dry Weight (lbf)", "RMC (Desired %)"="Relative Moisture (%)", "Tolerance(%)"="Tolerance (%)", "Measured IMC (lbs)"=w461) -> (w475:T25)
            n337 = call "Save File DPT RMC Calculations.vi"("Dryer IMC Data Input"=w475, "Error In"=w459) -> ("Dryer IMC Data Output"=w474:T25, "Error Out"=w466:errorcluster)  [unwired: 16 in]
            n338 = Unbundle By Name(w474) -> ("Minimum Weight (lbf)"=→"Minimum Weight (lbf)":dbl, "Average Weight (lbf)"=→"Average Weight (lbf)":dbl, "Maximum Weight (lbf)"=→"Maximum Weight (lbf)":dbl, "Actual Initial RMC (%)"=→"Measured Conent (%)":dbl, "Measured IMC In Range?"=w464:bool)
            n339 = Bundle By Name(cluster=w477, "Washer Controls In.Initialize.Washer In.Appliance Details.Dryer.Dryer Initial IMC Data"=w474) -> (w478:T42)
            n340 = case shown="True" w464 {
              tunnel: ["Out of Range" "In Range"] -> w465
              frame False {
              }
              frame True {
              }
            }
            n341 = local write "In Range?"(w465) -> ()
          }
          event "Bone Dry Weight (lbf)", "Relative Moisture (%)", "Tolerance (%)", "Measured Weight (lbf)": Value Change {
            n342 = event-data() -> ()  [unwired: 1 in, 6 out]
            n343 = local read "Bone Dry Weight (lbf)"() -> (w492:dbl)
            n344 = local read "Relative Moisture (%)"() -> (w493:dbl)
            n345 = local read "Tolerance (%)"() -> (w494:dbl)
            n346 = Unbundle By Name(w488) -> ("Washer Controls In.Initialize.Washer In.Appliance Details.Dryer.Dryer Initial IMC Data"=w491:T25)
            n347 = property on="Measured Weight (lbf)" class="DigNum (strict)"() -> ("Value"=w499:dbl)  [unwired: 2 in, 2 out]
            n348 = Bundle By Name(cluster=w491, "Bone Dry Wt(lbs)"=w492, "RMC (Desired %)"=w493, "Tolerance(%)"=w494, "Measured IMC (lbs)"=w499) -> (w490:T25)
            n349 = call "Save File DPT RMC Calculations.vi"("Dryer IMC Data Input"=w490, "Error In"=w485) -> ("Dryer IMC Data Output"=w489:T25, "Error Out"=w484:errorcluster)  [unwired: 16 in]
            n350 = Unbundle By Name(w489) -> ("Minimum Weight (lbf)"=w495:dbl, "Average Weight (lbf)"=w496:dbl, "Maximum Weight (lbf)"=w497:dbl, "Actual Initial RMC (%)"=w498:dbl, "Measured IMC In Range?"=w483:bool)
            n351 = Bundle By Name(cluster=w488, "Washer Controls In.Initialize.Washer In.Appliance Details.Dryer.Dryer Initial IMC Data"=w489) -> (w487:T42)
            n352 = case shown="True" w483 {
              tunnel: ["Out of Range" "In Range"] -> w482
              frame False {
              }
              frame True {
              }
            }
            "In Range?" <- w482
            n353 = local write "Minimum Weight (lbf)"(w495) -> ()
            n354 = local write "Average Weight (lbf)"(w496) -> ()
            n355 = local write "Maximum Weight (lbf)"(w497) -> ()
            n356 = local write "Measured Conent (%)"(w498) -> ()
          }
          event "Get Weigth": Value Change {
            n357 = event-data() -> ()  [unwired: 1 in, 6 out]
            n358 = Unbundle By Name(w503) -> ("Washer Controls In.Test Fixture Hardware.Weight Scale.Select Scale"=w502:string)
            n359 = case shown="\"IND560 SERIAL\"" w502 {
              tunnel: w503 -> [w511 w521]
              tunnel: [w513 w519] -> w507
              tunnel: w506 -> [w515 w518]
              tunnel: [w514 w517] -> w505
              tunnel: FALSE ("Use While Loop?") -> [w512 w516]
              frame "IND560 SERIAL" {
                n360 = Unbundle By Name(w511) -> ("Washer Controls In.Test Fixture Hardware.Weight Scale.Com Options.IND560Scale VISA"=w510:refnum<visa-resource-name>)
                n361 = call "IND560 Serial Tester.vi"("Use While Loop?"=w512, "Error In"=w515, "VISA Input"=w510) -> ("Error Out"=w514:errorcluster, "Net Weight"=w513:dbl)  [unwired: 7 in]
              }
              frame "GSE 350", Default {
                n362 = Unbundle By Name(w521) -> ("Washer Controls In.Test Fixture Hardware.Weight Scale.Com Options.GSE 350"=w520:refnum<visa-resource-name>)
                n363 = call "GSE 350 Main.vi"("Use While Loop?"=w516, "Error In"=w518, "VISA Refnum in"=w520) -> ("Error Out"=w517:errorcluster, "Weight (lb/kg)"=w519:dbl)  [unwired: 6 in, 1 out]
              }
            }
            n364 = local write "Cold Dryer Weigth"(w507) -> ()
            n365 = call <vilib>:"Clear Errors.vi"("error in (no error)"=w505) -> ("error out"=w508:errorcluster)  [unwired: 5 in, 1 out]
          }
          event Value Change {
            n366 = event-data() -> ("NewVal"=w522:T5)  [unwired: 1 in, 5 out]
            n367 = case shown="\"Other\"" w522 {
              frame "D2-Automatic Dryer", Default {
                n368 = property on="Cycles Per Year" class="DigNum (strict)"("Value"=283.0) -> ()  [unwired: 2 in, 2 out]
                n369 = property on="Moisture Reduction Factor" class="DigNum (strict)"("Value"=0.0) -> ()  [unwired: 2 in, 2 out]
                n370 = property on="Field Use Factor" class="DigNum (strict)"("Value"=0.0) -> ()  [unwired: 2 in, 2 out]
              }
              frame "D2-Timer Dryer" {
                n371 = property on="Cycles Per Year" class="DigNum (strict)"("Value"=283.0) -> ()  [unwired: 2 in, 2 out]
                n372 = property on="Moisture Reduction Factor" class="DigNum (strict)"("Value"=55.5) -> ()  [unwired: 2 in, 2 out]
                n373 = property on="Field Use Factor" class="DigNum (strict)"("Value"=1.18) -> ()  [unwired: 2 in, 2 out]
              }
              frame "D1-Automatic Dryer" {
                n374 = property on="Cycles Per Year" class="DigNum (strict)"("Value"=283.0) -> ()  [unwired: 2 in, 2 out]
                n375 = property on="Moisture Reduction Factor" class="DigNum (strict)"("Value"=53.5) -> ()  [unwired: 2 in, 2 out]
                n376 = property on="Field Use Factor" class="DigNum (strict)"("Value"=1.04) -> ()  [unwired: 2 in, 2 out]
              }
              frame "D1-Timer Dryer" {
                n377 = property on="Cycles Per Year" class="DigNum (strict)"("Value"=283.0) -> ()  [unwired: 2 in, 2 out]
                n378 = property on="Moisture Reduction Factor" class="DigNum (strict)"("Value"=53.5) -> ()  [unwired: 2 in, 2 out]
                n379 = property on="Field Use Factor" class="DigNum (strict)"("Value"=1.18) -> ()  [unwired: 2 in, 2 out]
              }
              frame "Other" {
                n380 = property on="Cycles Per Year" class="DigNum (strict)"("Value"=283.0) -> ()  [unwired: 2 in, 2 out]
                n381 = property on="Moisture Reduction Factor" class="DigNum (strict)"("Value"=0.0) -> ()  [unwired: 2 in, 2 out]
                n382 = property on="Field Use Factor" class="DigNum (strict)"("Value"=0.0) -> ()  [unwired: 2 in, 2 out]
              }
            }
            n383 = call <vilib>:"Add State(s) to Queue__jki_lib_state_machine.vi"("State(s) in (\"\")"=w524) -> ("States Out"=w525:string)  [unwired: 14 in]
          }
          event Panel Close? {
            # "Discard the event because we'll close the front panel ourselves in Macro: Exit"
            # "Close Panel button (pressed) Event\n(this executes Macro: Exit to terminate the VI)"
            n384 = event-data() -> ()  [unwired: 1 in, 1 out]
            n385 = call <vilib>:"Add State(s) to Queue__jki_lib_state_machine.vi"("State(s) in Front (\"\")"="Macro: Exit", "State(s) in (\"\")"=w547) -> ("States Out"=w546:string)  [unwired: 13 in]
            n386 = event-data("Discard?"=TRUE) -> ()  [unwired: 1 in, 1 out]
          }
        }
      }
      frame "---------- Core ----------" {
        n387 = call <vilib>:"Add State(s) to Queue__jki_lib_state_machine.vi"("State(s) in (\"\")"=w551) -> ("States Out"=w550:string)  [unwired: 14 in]
      }
      frame Default {
        w561 = 42 items=["No error", "Argument error", "Memory is full", "Out of zone", "End of file", "File already open", "Generic file I/O error", "File not found", "File permission error", "Disk is full", "Duplicate path", "Too many files open", "System feature not enabled", "Resource file not found", "Cannot add resource", "Resource not found", "Image not found", "Image memory error", "Pen does not exist", "Config type invalid", "Config token not found", "Config parse error", "Config memory error", "Bad external code format", "Bad external code offset", "External code not present", "Null window", "Destroy window error", "Null menu", "Print aborted", "Bad print record", "Print driver error", "Windows error during printing", "Memory error during printing", "Print dialog error", "Generic print error", "Invalid device refnum", "Device not found", "Device parameter error", "Device unit error", "Cannot open device", "Device call aborted", "Generic error", "Cancelled by user", "Object ID too low", "Object ID too high", "Object not in heap", "Unknown heap", "Unknown object (invalid DefProc)", "Unknown object (DefProc not in table)", "Message out of range", "Invalid (null) method", "Unknown message", "Manager call not supported", "Bad address", "Network operation in progress", "Network operation timed out", "Connection is busy", "Network attribute not supported", "Network error", "Address in use", "System out of memory", "Connection aborted", "Connection refused", "Not connected", "Already connected", "Connection closed", "Initialization error (interapplication manager)", "Bad occurrence", "Wait on unbound occurrence handler", "Occurrence queue overflow", "Datalog type conflict", "Unused", "Unrecognized type (interapplication manager)", "Memory corrupt", "Failed to make temporary DLL", "Old CIN version", "Drag socket not found", "Failed to load drop-object", "Failed to register OLE object", "Failed to release OLE object", "Format specifier type mismatch", "Unknown format specifier", "Too few format specifiers", "Too many format specifiers", "Scan failed", "Newer CIN version", "Error converting to variant", "Runtime menu error", "Password tampered", "Variant attribute not found", "Incompatible variant data type", "Event data is not available", "Event Store is not present", "Occurrence is not found", "Event Queue is not created", "Event info is not available", "Refnum passed is NULL", "Error retrieving Class GUID", "Error retrieving CoClass GUID", "Error retrieving TypeLib GUID.", "Bad built application magic bytes.", "Specific driver is different from the specific driver associated with the Logical Name.", "There is no session opened to the class driver.", "Max Error", "MAX - Error with config objects", "MAX - Error loading configuration", "MAX - Group not supported"]
        # "Current State"
        # "Handle mistyped state name (developer tool)"
        n388 = Format Into String(format string="Software Exception: Unhandled State \"%s\"." ("message"), error in=w557, w552) -> (resulting string=w560:string, error out=w559:errorcluster)  [unwired: 1 in]
        n389 = call <vilib>:"Error Cluster From Error Code.vi"("show call chain? (False)"=TRUE, "error in (no error)"=w559, "error message (\"\")"=w560, "error code (0)"=w561) -> ("error out"=w558:errorcluster)  [unwired: 5 in]
        n390 = call <vilib>:"Add State(s) to Queue__jki_lib_state_machine.vi"("State(s) in (\"\")"=w556) -> ("States Out"=w555:string)  [unwired: 14 in]
      }
      frame "Initialize Core Data" {
        # "originally closed?"
        # "exe?"
        # "If panel starts closed or is an EXE, then close it when we exit"
        n391 = property class="VI"() -> ("Front Panel.Open"=w571:bool)  [unwired: 2 in, 2 out]
        n392 = property class="App"() -> ("App.Kind"=w570:T28)  [unwired: 2 in, 2 out]
        n393 = control-ref of="Current VI Reference"() -> (w564:refnum<vi>)
        n394 = Not(x=w571) -> (.not. x?=w568:bool)
        n395 = Equal?(x=w570, y=T28."Run Time System" ("Application:Kind")) -> (x = y?=w567:bool)
        n396 = Or(x=w568, y=w567) -> (x .or. y?=w565:bool)
        n397 = Bundle By Name(cluster=w566, "Core.Current VI Reference"=w564, "Core.Close Panel on Exit?"=w565) -> (w572:T42)
        n398 = call <vilib>:"Add State(s) to Queue__jki_lib_state_machine.vi"("State(s) in (\"\")"=w574) -> ("States Out"=w573:string)  [unwired: 14 in]
      }
      frame "Error Handler" {
        # "Unhandled Error -- Display it"
        # "Handle any errors here.\nYou can also output any states to clean-up after errors occur"
        # "Clear error"
        n399 = call <vilib>:"General Error Handler.vi"("error in (no error)"=w579) -> ()  [unwired: 10 in, 5 out]
        n400 = Bundle By Name(cluster=w577, "Error Flag"=TRUE) -> (w576:T42)
        n401 = call <vilib>:"Add State(s) to Queue__jki_lib_state_machine.vi"("State(s) in Front (\"\")"="Macro: Exit", "State(s) in (\"\")"=w582) -> ("States Out"=w581:string)  [unwired: 13 in]
        "Unhandled Error" <- w579
      }
      frame "Exit" {
        n402 = call <vilib>:"Add State(s) to Queue__jki_lib_state_machine.vi"("State(s) in (\"\")"=w587) -> ("States Out"=w586:string)  [unwired: 14 in]
      }
      frame "---------- Data ----------" {
        n403 = call <vilib>:"Add State(s) to Queue__jki_lib_state_machine.vi"("State(s) in (\"\")"=w591) -> ("States Out"=w590:string)  [unwired: 14 in]
      }
      frame "Data: Initialize" {
        w595 = T41 {"Manufacturer-Dish (Array):"=[], "Unit Control-Dish (Array):"=[], "Test Type (Array):"=[], "Cycle Mode-Dish(Array): "=[], "Inlet Temperature (F)-Dish (Array):"=[], "Detergent-Dish (Array):"=[], "Cycle Selection (Array):"=[], "Wash Temperature (Array):"=[], "Rinse Temperature (Array):"=[], "Load Size (Array):"=[], "Water Pressure (PSI) (Array) :"=[], "Ambient RH (Array):"=[], "Supply Voltage (Array):"=[], "Station ID (Array):"=[], "Lab ID (Array):"=[], "TR Number (Array):"=[], "Cold Water Temperature (Fahrenheit) (Array):"=[], "Technician (Array):"=[], "Frequency (Array):"=[], "Build (Array):"=[], "Hot Water Temperature (Fahrenheit) (Array):"=[], "Heating Mode (Array):"=[], "Ambient Temperature (F) (Array):"=[], "Dryer Type (Array):"=[], "Exhaust (Array):"=[], "Drying Cycle (Array):"=[], "Heat Setting (Array):"=[], "Dryness Setting (Array):"=[], "Nominal Load Weigth (lbs) (Array):"=[], "Load Type (Array):"=[]}  # Drop Down Controls
        w598 = T43 {"Current VI Reference"=refnum, "Close Panel on Exit?"=FALSE}  # Core
        w599 = FALSE  # Error Flag
        n404 = local write "Program Tab"(T1."Main" ("Program Tab")) -> ()
        n405 = call <vilib>:"Add State(s) to Queue__jki_lib_state_machine.vi"("State(s) in (\"\")"=w603) -> ("States Out"=w602:string)  [unwired: 14 in]
        n406 = Unbundle By Name("Washer Controls In") -> ("Initialize.Washer In.Appliance Details.Appliance Common.Cycles Per Year"=w593:u32)
        n407 = Bundle("Core"=w598, "Error Flag"=w599, "Washer Controls In"="Washer Controls In", "LV Program"="LV Program", "Filepath In"="Filepath In", "Drop Down Controls"=w595) -> (w601:T42)  [unwired: 1 in]
        n408 = property on="Cycles Per Year" class="DigNum (strict)"("Value"=w593) -> ()  [unwired: 2 in, 2 out]
      }
      frame "Load Configuration" {
        # "This prevents overwriting data that is already good.\n\nLoad the config file...then open the front panel"
        # "Update with correct info"
        n409 = Unbundle By Name(w615) -> ("Washer Controls In.Test Fixture Hardware"=w608:T13, "LV Program"=w612:T9, "Filepath In.General Setup Paths.File Save Configuration Data Path"=w606:path)
        n410 = call "Save File DOE Configuration.vi"("Add/Remove Enum"=T27."Load Standard", "error in (no error)"=w617, "File Save Configuration Data Path"=w606) -> ("error out"=w618:errorcluster, "Full Data Output"=w611:string[][])  [unwired: 6 in, 1 out]
        n411 = call "Save File DOE Extract Configuration Data.vi"("Test Fixture Hardware"=w608, "LV Program"=w612, "Input Config Files"=w611) -> ("Drop Down Core Output"=w614:T44, "Test Fixture Hardware Output"=w613:T13, "Filepath Output"=w605:T10)  [unwired: 6 in]
        n412 = Unbundle By Name(w605) -> ("General Setup Paths.Data Folder Path"=w604:path)
        n413 = Unbundle By Name(w614) -> ("Drop Down Controls"=w609:T41)
        n414 = case shown="\"Open Front Panel\"" w607 {
          tunnel: w615 -> [w624 w629]
          tunnel: w613 -> [_ w628]
          tunnel: [w623 w627] -> w610
          tunnel: w609 -> [w622 w626]
          tunnel: w604 -> [w621 w625]
          frame "Open Front Panel" {
            n415 = Bundle By Name(cluster=w624, "Filepath In.General Setup Paths.Data Folder Path"=w621, "Drop Down Controls"=w622) -> (w623:T42)
          }
          frame Default {
            n416 = Bundle By Name(cluster=w629, "Filepath In.General Setup Paths.Data Folder Path"=w625, "Washer Controls In.Test Fixture Hardware"=w628, "Drop Down Controls"=w626) -> (w627:T42)
          }
        }
        n417 = call <vilib>:"Add State(s) to Queue__jki_lib_state_machine.vi"("State(s) in (\"\")"=w620) -> ("States Out"=w619:string)  [unwired: 14 in]
      }
      frame "Populate Controls" {
        # "Update with correct info"
        n418 = Unbundle By Name(w639) -> ("Drop Down Controls.Manufacturer-Dish (Array):"=w660:string[], "Drop Down Controls.Unit Control-Dish (Array):"=w659:string[], "Drop Down Controls.Test Type (Array):"=w658:string[], "Drop Down Controls.Cycle Mode-Dish(Array):"=w657:string[], "Drop Down Controls.Inlet Temperature (F)-Dish (Array):"=w656:string[], "Drop Down Controls.Detergent-Dish (Array):"=w655:string[], "Drop Down Controls.Cycle Selection (Array):"=w654:string[], "Drop Down Controls.Wash Temperature (Array):"=w653:string[], "Drop Down Controls.Rinse Temperature (Array):"=w652:string[], "Drop Down Controls.Load Size (Array):"=w651:string[], "Drop Down Controls.Water Pressure (PSI) (Array) :"=w650:string[], "Drop Down Controls.Ambient RH (Array):"=w649:string[], "Drop Down Controls.Supply Voltage (Array):"=w648:string[], "Drop Down Controls.Station ID (Array):"=w640:string[], "Drop Down Controls.Lab ID (Array):"=w647:string[], "Drop Down Controls.TR Number (Array):"=w646:string[], "Drop Down Controls.Cold Water Temperature (Fahrenheit) (Array):"=w645:string[], "Drop Down Controls.Technician (Array):"=w644:string[], "Drop Down Controls.Frequency (Array):"=w643:string[], "Drop Down Controls.Build (Array):"=w642:string[], "Drop Down Controls.Hot Water Temperature (Fahrenheit) (Array):"=w641:string[], "Drop Down Controls.Heating Mode (Array):"=w638:string[], "Drop Down Controls.Ambient Temperature (F) (Array):"=w637:string[], "Drop Down Controls.Dryer Type (Array):"=w636:string[], "Drop Down Controls.Exhaust (Array):"=w635:string[], "Drop Down Controls.Drying Cycle (Array):"=w634:string[], "Drop Down Controls.Heat Setting (Array):"=w633:string[], "Drop Down Controls.Dryness Setting (Array):"=w632:string[], "Drop Down Controls.Nominal Load Weigth (lbs) (Array):"=w631:string[], "Drop Down Controls.Load Type (Array):"=w630:string[])
        n419 = property on="Manufacturer-Dish:" class="CmbBox"("Strings[]"=w660) -> ()  [unwired: 2 in, 2 out]
        n420 = property on="Unit Control-Dish:" class="CmbBox"("Strings[]"=w659) -> ()  [unwired: 2 in, 2 out]
        n421 = property on="Test Type:" class="CmbBox"("Strings[]"=w658) -> ()  [unwired: 2 in, 2 out]
        n422 = property on="Cycle Mode-Dish:" class="CmbBox"("Strings[]"=w657) -> ()  [unwired: 2 in, 2 out]
        n423 = property on="Inlet Temperature-Dish:" class="CmbBox"("Strings[]"=w656) -> ()  [unwired: 2 in, 2 out]
        n424 = property on="Detergent-Dish:" class="CmbBox"("Strings[]"=w655) -> ()  [unwired: 2 in, 2 out]
        n425 = property on="Cycle Selection" class="CmbBox"("Strings[]"=w654) -> ()  [unwired: 2 in, 2 out]
        n426 = property on="Wash Temperature" class="CmbBox"("Strings[]"=w653) -> ()  [unwired: 2 in, 2 out]
        n427 = property on="Rinse Temperature" class="CmbBox"("Strings[]"=w652) -> ()  [unwired: 2 in, 2 out]
        n428 = property on="Load Size" class="CmbBox"("Strings[]"=w651) -> ()  [unwired: 2 in, 2 out]
        n429 = property on="Water Pressure (PSI):" class="CmbBox"("Strings[]"=w650) -> ()  [unwired: 2 in, 2 out]
        n430 = property on="Ambient RH:" class="CmbBox"("Strings[]"=w649) -> ()  [unwired: 2 in, 2 out]
        n431 = property on="Supply Voltage:" class="CmbBox"("Strings[]"=w648) -> ()  [unwired: 2 in, 2 out]
        n432 = property on="Station ID:" class="CmbBox"("Strings[]"=w640) -> ()  [unwired: 2 in, 2 out]
        n433 = property on="Lab ID:" class="CmbBox"("Strings[]"=w647) -> ()  [unwired: 2 in, 2 out]
        n434 = property on="TR Number:" class="CmbBox"("Strings[]"=w646) -> ()  [unwired: 2 in, 2 out]
        n435 = property on="Cold Water Temperature (Fahrenheit)" class="CmbBox"("Strings[]"=w645) -> ()  [unwired: 2 in, 2 out]
        n436 = property on="Technician:" class="CmbBox"("Strings[]"=w644) -> ()  [unwired: 2 in, 2 out]
        n437 = property on="Frequency:" class="CmbBox"("Strings[]"=w643) -> ()  [unwired: 2 in, 2 out]
        n438 = property on="Build:" class="CmbBox"("Strings[]"=w642) -> ()  [unwired: 2 in, 2 out]
        n439 = property on="Hot Water Temperature (Fahrenheit)" class="CmbBox"("Strings[]"=w641) -> ()  [unwired: 2 in, 2 out]
        n440 = property on="Heating Mode" class="CmbBox (strict)"("Strings[]"=w638) -> ()  [unwired: 2 in, 2 out]
        n441 = property on="Ambient Temperature (F):" class="CmbBox"("Strings[]"=w637) -> ()  [unwired: 2 in, 2 out]
        n442 = property on="Dryer Type:" class="CmbBox"("Strings[]"=w636) -> ()  [unwired: 2 in, 2 out]
        n443 = property on="Exhaust:" class="CmbBox"("Strings[]"=w635) -> ()  [unwired: 2 in, 2 out]
        n444 = property on="Drying Cycle:" class="CmbBox"("Strings[]"=w634) -> ()  [unwired: 2 in, 2 out]
        n445 = property on="Heat Setting:" class="CmbBox"("Strings[]"=w633) -> ()  [unwired: 2 in, 2 out]
        n446 = property on="Dryness Setting:" class="CmbBox"("Strings[]"=w632) -> ()  [unwired: 2 in, 2 out]
        n447 = property on="Nominal Load Weight (lbs):" class="CmbBox"("Strings[]"=w631) -> ()  [unwired: 2 in, 2 out]
        n448 = property on="Load Type:" class="CmbBox"("Strings[]"=w630) -> ()  [unwired: 2 in, 2 out]
        n449 = call <vilib>:"Add State(s) to Queue__jki_lib_state_machine.vi"("State(s) in (\"\")"=w663) -> ("States Out"=w662:string)  [unwired: 14 in]
      }
      frame "Data: Cleanup" {
        n450 = Unbundle By Name(w664) -> ("Core.Current VI Reference"=w667:refnum<vi>)
        n451 = Close Reference(reference=w667, error in (no error)=w666) -> (error out=w665:errorcluster)
        n452 = call <vilib>:"Add State(s) to Queue__jki_lib_state_machine.vi"("State(s) in (\"\")"=w669) -> ("States Out"=w668:string)  [unwired: 14 in]
      }
      frame "---------- UI ----------" {
        n453 = call <vilib>:"Add State(s) to Queue__jki_lib_state_machine.vi"("State(s) in (\"\")"=w673) -> ("States Out"=w672:string)  [unwired: 14 in]
      }
      frame "UI: Initialize" {
        n454 = Unbundle By Name(w686) -> ("LV Program"=w685:T9, "Filepath In.General Setup Paths.Tool Base Path"=w677:path)
        n455 = case shown="Default" w685 {
          tunnel: [w695 w696 w697 w698] -> w684
          tunnel: [w695 w696 w697 w698] -> w683
          frame Default {
            w695 = FALSE ("Visible")
          }
          frame "Dishwasher Kitchen" {
            w696 = FALSE ("Visible")
          }
          frame "Portable Stand" {
            w697 = FALSE ("Visible")
          }
          frame "HEWH", "PRAT", "HEWH RLT" {
            w698 = TRUE ("Visible")
          }
        }
        n456 = Current VI's Path() -> (path=w692:path)
        n457 = call "UTILITY This VIs Path.vi"("path"=w692) -> ("FileVersionInfo Out"=w687:T23)  [unwired: 8 in, 6 out]
        n458 = Format Date/Time String(time format string (%c)="Date_%m_%d_%Y_Time_%H_%M") -> (date/time string=w690:string)  [unwired: 2 out]
        n459 = call "UTILITY IP and Computer Name.vi"() -> ("IP Address"=w688:string, "Computer Name"=w689:string)  [unwired: 10 in]
        n460 = property on="Get Model Number" class="Bool"("Visible"=w684) -> ()  [unwired: 2 in, 2 out]
        n461 = property on="Get Serial Number" class="Bool"("Visible"=w683) -> ()  [unwired: 2 in, 2 out]
        n462 = call "Save File General Main File Save Configuration Path.vi"("Error In"=w676, "Tool Base Path"=w677) -> ("Error Out"=w682:errorcluster, "Appliance Previous Run Path"=w679:path, "Calibration File Path"=w680:path, "File Save Configuration Data Path"=w681:path, "DOE Capacity Path"=w678:path)  [unwired: 5 in]
        n463 = Bundle By Name(cluster=w686, "Washer Controls In.Initialize.Washer In.Appliance Details.FileVersionInfo"=w687, "Washer Controls In.Initialize.Washer In.Appliance Details.Appliance Common.Test Date:"=w690, "Washer Controls In.Initialize.Washer In.Appliance Details.Appliance Common.Computer Name:"=w689, "Washer Controls In.Initialize.Washer In.Appliance Details.Appliance Common.IP Address:"=w688, "Filepath In.General Setup Paths.DOE Capacity Path"=w678, "Filepath In.General Setup Paths.File Save Configuration Data Path"=w681, "Filepath In.General Setup Paths.Calibration File Path"=w680, "Filepath In.General Setup Paths.File Save Previous Run Path"=w679) -> (w675:T42)
        n464 = Unbundle By Name(w675) -> ("Filepath In"=w674:T10)
        n465 = local write "Filepath In"(w674) -> ()
        n466 = call <vilib>:"Add State(s) to Queue__jki_lib_state_machine.vi"("State(s) in (\"\")"=w694) -> ("States Out"=w693:string)  [unwired: 14 in]
      }
      frame "UI: Cursor Set" {
        # "Argument"
        # "Set and Unset Cursor Busy.\n(Usage: \"UI: Cursor Set >> Busy|Idle\")"
        n467 = case shown="\"Idle\", Default" w699 {
          tunnel: w701 -> [w706 w708]
          tunnel: [w705 w707] -> w700
          frame "Idle", Default {
            n468 = call <vilib>:"Unset Busy.vi"("error in (no error)"=w706) -> ("error out"=w705:errorcluster)  [unwired: 10 in]
          }
          frame "Busy" {
            n469 = call <vilib>:"Set Busy.vi"("error in (no error)"=w708) -> ("error out"=w707:errorcluster)  [unwired: 9 in, 1 out]
          }
        }
        n470 = call <vilib>:"Add State(s) to Queue__jki_lib_state_machine.vi"("State(s) in (\"\")"=w704) -> ("States Out"=w703:string)  [unwired: 14 in]
      }
      frame "UI: Front Panel State" {
        # "Argument"
        # "Set Front Panel Open or Closed\n(Usage: \"UI: Front Panel State >> Open|Close\")"
        n471 = Unbundle By Name(w711) -> ("Core.Current VI Reference"=w710:refnum<vi>)
        n472 = case shown="\"Open\", Default" w709 {
          tunnel: w713 -> [w719 w732]
          tunnel: [w721 w733] -> w712
          tunnel: w710 -> [w720 w730]
          frame "Open", Default {
            n473 = property class="VI"(reference=w720, error in=w719) -> (reference out=w717:refnum<vi>, error out=w718:errorcluster, "Front Panel.Open"=w716:bool)
            n474 = case shown="True" w716 {
              tunnel: [w724 w727] -> w721
              tunnel: w718 -> [w723 w727]
              tunnel: w717 -> [w722 _]
              frame False {
                n475 = invoke class="VI" method="FP.Open"(reference=w722, error in=w723, "Activate"=TRUE, "State"=T29."Standard") -> (error out=w724:errorcluster)  [unwired: 1 in, 4 out]
              }
              frame True {
              }
            }
          }
          frame "Close" {
            n476 = property class="VI"(reference=w730, error in=w732) -> (reference out=w729:refnum<vi>, error out=w731:errorcluster, "Front Panel.Open"=w728:bool)
            n477 = case shown="True" w728 {
              tunnel: [w734 w737] -> w733
              tunnel: w731 -> [w734 w736]
              tunnel: w729 -> [_ w735]
              frame False {
              }
              frame True {
                n478 = invoke class="VI" method="FP.Close"(reference=w735, error in=w736) -> (error out=w737:errorcluster)  [unwired: 1 in, 2 out]
              }
            }
          }
        }
        n479 = call <vilib>:"Add State(s) to Queue__jki_lib_state_machine.vi"("State(s) in (\"\")"=w715) -> ("States Out"=w714:string)  [unwired: 14 in]
      }
      frame "---------- Macro ----------" {
        n480 = call <vilib>:"Add State(s) to Queue__jki_lib_state_machine.vi"("State(s) in (\"\")"=w741) -> ("States Out"=w740:string)  [unwired: 14 in]
      }
      frame "Macro: Initialize" {
        n481 = property on="OK" class="Bool"("Key Focus"=FALSE) -> ()  [unwired: 2 in, 2 out]
        n482 = local write "Build:"("" ("Dryer Type:")) -> ()
        n483 = call <vilib>:"Add State(s) to Queue__jki_lib_state_machine.vi"("State(s) in Front (\"\")"="Data: Initialize\nInitialize Core Data\nUI: Initialize", "State(s) in (\"\")"=w748) -> ("States Out"=w747:string)  [unwired: 13 in]
      }
      frame "Macro: Exit" {
        n484 = Unbundle By Name(w755) -> ("Core.Close Panel on Exit?"=w749:bool)
        n485 = Select(t="UI: Front Panel State >> Close", s=w749, f="") -> (s? t:f=w752:string)
        n486 = call <vilib>:"Add State(s) to Queue__jki_lib_state_machine.vi"("State(s) in (\"\")"=w752, "State(s) at Back (\"\")"="Data: Cleanup\nExit") -> ("States Out"=w750:string)  [unwired: 13 in]
        n487 = call <vilib>:"Add State(s) to Queue__jki_lib_state_machine.vi"("State(s) in Front (\"\")"=w750, "State(s) in (\"\")"=w758) -> ("States Out"=w757:string)  [unwired: 13 in]
      }
      frame "---------- New Category ----------" {
        n488 = call <vilib>:"Add State(s) to Queue__jki_lib_state_machine.vi"("State(s) in (\"\")"=w762) -> ("States Out"=w761:string)  [unwired: 14 in]
      }
      frame "Get Main Info" {
        n489 = Equal?(x="Station ID:", y="Select Room/Stall") -> (x = y?=w765:bool)
        n490 = case shown="False" w765 {
          tunnel: "Station ID:" -> [w787 _]
          tunnel: [w787 w788] -> w763
          frame False {
          }
          frame True {
            w788 = ""
            n491 = local write "Station ID:"(w788) -> ()
          }
        }
        n492 = Bundle By Name(cluster=w782, "Washer Controls In.Initialize.Washer In.Appliance Details.Appliance Common.TR Number:"="TR Number:", "Washer Controls In.Initialize.Washer In.Appliance Details.Appliance Common.Lab ID:"="Lab ID:", "Washer Controls In.Initialize.Washer In.Appliance Details.Appliance Common.Model Number:"="Model:", "Washer Controls In.Initialize.Washer In.Appliance Details.Appliance Common.Serial Number:"="Serial Number:", "Washer Controls In.Initialize.Washer In.Display Data (RLT).Serial Number Display"="Serial Number:", "Washer Controls In.Initialize.Washer In.Appliance Details.Appliance Common.Station ID:"=w763, "Washer Controls In.Initialize.Washer In.Display Data (RLT).Station Label Display"=w763, "Washer Controls In.Initialize.Washer In.Appliance Details.Appliance Common.Engineer:"="Engineer:", "Washer Controls In.Initialize.Washer In.Appliance Details.Appliance Common.Technician:"="Technician:", "Washer Controls In.Initialize.Washer In.Appliance Details.Appliance Common.Water Pressure (PSI):"="Water Pressure (PSI):", "Washer Controls In.Initialize.Washer In.Appliance Details.Appliance Common.Ambient RH:"="Ambient RH:", "Washer Controls In.Initialize.Washer In.Appliance Details.Appliance Common.Ambient Temperature (F):"="Ambient Temperature (F):", "Washer Controls In.Initialize.Washer In.Appliance Details.Appliance Common.Voltage:"="Supply Voltage:", "Washer Controls In.Initialize.Washer In.Appliance Details.Appliance Common.Frequency:"="Frequency:", "Washer Controls In.Initialize.Washer In.Appliance Details.Appliance Common.Build:"="Build:", "Washer Controls In.Initialize.Washer In.Appliance Details.Appliance Common.Comments:"="Comments:", "Washer Controls In.Initialize.Washer In.Appliance Details.Appliance Common.Test Type:"="Test Type:", "Washer Controls In.Initialize.Washer In.Appliance Details.Appliance Common.Load Run #:"="Load Run #:") -> (w784:T42)
        n493 = call <vilib>:"Add State(s) to Queue__jki_lib_state_machine.vi"("State(s) in (\"\")"=w783) -> ("States Out"=w786:string)  [unwired: 14 in]
      }
      frame "Check Contents" {
        # "If all of the data fields have information go ahead and generate the filename"
        n494 = Unbundle By Name(w801) -> ("Washer Controls In.Initialize.Washer In.Appliance Details.Appliance Common.TR Number:"=w799:string, "Washer Controls In.Initialize.Washer In.Appliance Details.Appliance Common.Lab ID:"=w798:string, "Washer Controls In.Initialize.Washer In.Appliance Details.Appliance Common.Serial Number:"=w797:string, "Washer Controls In.Initialize.Washer In.Appliance Details.Appliance Common.Station ID:"=w796:string, "Washer Controls In.Initialize.Washer In.Appliance Details.Dryer.Dryer Initial IMC Data.Measured IMC In Range?"=w793:bool, "LV Program"=w789:T9)
        n495 = Build Array(w799, w798, w797, w796) -> (w795:string[])
        n496 = for {
          tunnel: w795 -> [w813] mode=indexing
          tunnel: [w812] -> w794 mode=indexing
          n497 = String Length(string=w813) -> (length=w814:i32)
          n498 = Greater Than 0?(x=w814) -> (x > 0?=w812:bool)
        }
        n499 = And Array Elements(Boolean array=w794) -> (logical AND=w791:bool)
        n500 = case shown="Default" w789 {
          tunnel: w793 -> [_ w809]
          tunnel: ["You Must ENTER the following:\n1. TR Number                 \n2. Lab ID                          \n3. Serial Number            \n4. Station ID                    " ("message") "You Must ENTER the following:\n1. TR Number \n2. Lab ID \n3. Serial Number\n4. Station ID\n5. Initial Moisure Content Info                    " ("message")] -> w792
          tunnel: w791 -> [w806 w810]
          tunnel: [w806 w808] -> w790
          frame Default {
          }
          frame "Dryer" {
            n501 = And(x=w810, y=w809) -> (x .and. y?=w808:bool)
          }
        }
        n502 = case shown="True" w790 {
          tunnel: ["" w818] -> w802
          tunnel: w801 -> [w816 w820]
          tunnel: [w816 w820] -> w800
          tunnel: w789 -> [_ w819]
          tunnel: w792 -> [w815 _]
          frame False {
            n503 = One Button Dialog(message=w815) -> ()  [unwired: 1 in, 1 out]
          }
          frame True {
            n504 = case shown="\"DOE Stand\", \"Portable Stand\", Default" w819 {
              tunnel: ["Get Washer Info\nGenerate Filename\nGenerate Header Data" "Get Dish Info\nGenerate Filename\nGenerate Header Data" "Get HEWH Info\nGenerate Filename\nGenerate Header Data" "Get Dryer Info\nGenerate Filename\nGenerate Header Data" "Get Refrigeration\nGenerate Filename\nGenerate Header Data"] -> w818
              frame "DOE Stand", "Portable Stand", Default {
              }
              frame "Dishwasher Kitchen" {
              }
              frame "HEWH", "PRAT", "HEWH RLT" {
              }
              frame "Dryer" {
              }
              frame "Refrigeration" {
              }
            }
          }
        }
        n505 = call <vilib>:"Add State(s) to Queue__jki_lib_state_machine.vi"("State(s) in Front (\"\")"=w802, "State(s) in (\"\")"=w805) -> ("States Out"=w804:string)  [unwired: 13 in]
      }
      frame "Get Dish Info" {
        n506 = Unbundle By Name(w834) -> ("LV Program"=w833:T9)
        n507 = case shown="\"DOE Stand\", \"Portable Stand\", Default" w833 {
          tunnel: w834 -> [w839 w848 w849 w850]
          tunnel: [w839 w847 w849 w850] -> w836
          tunnel: "Manufacturer-Dish:" -> [_ w846 _ _]
          tunnel: "Unit Control-Dish:" -> [_ w845 _ _]
          tunnel: "Cycle Mode-Dish:" -> [_ w844 _ _]
          tunnel: "Inlet Temperature-Dish:" -> [_ w843 _ _]
          tunnel: "Detergent-Dish:" -> [_ w842 _ _]
          tunnel: "Auto Cup Weight (gm):" -> [_ w841 _ _]
          tunnel: "Open Cup Weight (gm):" -> [_ w840 _ _]
          frame "DOE Stand", "Portable Stand", Default {
          }
          frame "Dishwasher Kitchen" {
            n508 = Bundle By Name(cluster=w848, "Washer Controls In.Initialize.Washer In.Appliance Details.Dishwasher Info.Manufacturer-Dish:"=w846, "Washer Controls In.Initialize.Washer In.Appliance Details.Dishwasher Info.Unit Control-Dish:"=w845, "Washer Controls In.Initialize.Washer In.Appliance Details.Dishwasher Info.Cycle Mode-Dish:"=w844, "Washer Controls In.Initialize.Washer In.Appliance Details.Dishwasher Info.Inlet Temperature-Dish:"=w843, "Washer Controls In.Initialize.Washer In.Appliance Details.Dishwasher Info.Detergent-Dish:"=w842, "Washer Controls In.Initialize.Washer In.Appliance Details.Dishwasher Info.Auto Cup Weight (gm):"=w841, "Washer Controls In.Initialize.Washer In.Appliance Details.Dishwasher Info.Open Cup Weight (gm):"=w840) -> (w847:T42)
          }
          frame "HEWH", "PRAT", "HEWH RLT" {
          }
          frame "Dryer" {
          }
        }
        n509 = call <vilib>:"Add State(s) to Queue__jki_lib_state_machine.vi"("State(s) in (\"\")"=w835) -> ("States Out"=w838:string)  [unwired: 14 in]
      }
      frame "Get Washer Info" {
        n510 = Unbundle By Name(w864) -> ("LV Program"=w863:T9)
        n511 = case shown="\"DOE Stand\", \"Portable Stand\", Default" w863 {
          tunnel: w864 -> [w882 w883 w884 w885]
          tunnel: [w881 w883 w884 w885] -> w866
          tunnel: "Model Family" -> [w880 _ _ _]
          tunnel: "Program Name" -> [w879 _ _ _]
          tunnel: "Cycle Selection" -> [w878 _ _ _]
          tunnel: "Wash Temperature" -> [w877 _ _ _]
          tunnel: "Rinse Temperature" -> [w876 _ _ _]
          tunnel: "Load Size" -> [w875 _ _ _]
          tunnel: "Hot Water Temperature (Fahrenheit)" -> [w874 _ _ _]
          tunnel: "Cold Water Temperature (Fahrenheit)" -> [w873 _ _ _]
          tunnel: "Capacity (cu.ft)" -> [w872 _ _ _]
          tunnel: "Initial Cloth Weight:" -> [w871 _ _ _]
          tunnel: "Cloth Lot:" -> [w870 _ _ _]
          tunnel: "Unit Type Display" -> [w869 _ _ _]
          frame "DOE Stand", "Portable Stand", Default {
            n512 = Bundle By Name(cluster=w882, "Washer Controls In.Initialize.Washer In.Appliance Details.Washer Info.Model Family:"=w880, "Washer Controls In.Initialize.Washer In.Appliance Details.Washer Info.Program Name:"=w879, "Washer Controls In.Initialize.Washer In.Appliance Details.Washer Info.Cycle Selection:"=w878, "Washer Controls In.Initialize.Washer In.Appliance Details.Washer Info.Wash Temperature:"=w877, "Washer Controls In.Initialize.Washer In.Appliance Details.Washer Info.Rinse Temperature:"=w876, "Washer Controls In.Initialize.Washer In.Appliance Details.Washer Info.Load Size:"=w875, "Washer Controls In.Initialize.Washer In.Appliance Details.Washer Info.Hot Water Temperature (Fahrenheit):"=w874, "Washer Controls In.Initialize.Washer In.Appliance Details.Washer Info.Cold Water Temperature (Fahrenheit):"=w873, "Washer Controls In.Initialize.Washer In.Appliance Details.Washer Info.Capacity (cu.ft):"=w872, "Washer Controls In.Initialize.Washer In.Appliance Details.Washer Info.Initial Cloth Weight:"=w871, "Washer Controls In.Initialize.Washer In.Appliance Details.Washer Info.Cloth Lot:"=w870, "Washer Controls In.Initialize.Washer In.Display Data (RLT).Unit Type Display"=w869) -> (w881:T42)
          }
          frame "Dishwasher Kitchen" {
          }
          frame "HEWH", "PRAT", "HEWH RLT" {
          }
          frame "Dryer" {
          }
        }
        n513 = call <vilib>:"Add State(s) to Queue__jki_lib_state_machine.vi"("State(s) in (\"\")"=w865) -> ("States Out"=w868:string)  [unwired: 14 in]
      }
      frame "Get HEWH Info" {
        n514 = Unbundle By Name(w888) -> ("LV Program"=w887:T9)
        n515 = case shown="\"HEWH\", \"PRAT\", \"HEWH RLT\"" w887 {
          tunnel: w888 -> [w893 w894 w897 w898]
          tunnel: [w893 w894 w896 w898] -> w890
          tunnel: "Heating Mode" -> [_ _ w895 _]
          frame "DOE Stand", "Portable Stand", Default {
          }
          frame "Dishwasher Kitchen" {
          }
          frame "HEWH", "PRAT", "HEWH RLT" {
            n516 = Bundle By Name(cluster=w897, "Washer Controls In.Initialize.Washer In.Appliance Details.Water Heater.Heating Mode:"=w895) -> (w896:T42)
          }
          frame "Dryer" {
          }
        }
        n517 = call <vilib>:"Add State(s) to Queue__jki_lib_state_machine.vi"("State(s) in (\"\")"=w889) -> ("States Out"=w892:string)  [unwired: 14 in]
      }
      frame "Get Dryer Info" {
        n518 = Unbundle By Name(w914) -> ("LV Program"=w913:T9)
        n519 = case shown="\"Dryer\"" w913 {
          tunnel: w914 -> [w919 w920 w921 w937]
          tunnel: [w919 w920 w921 w936] -> w916
          tunnel: "Heat Setting:" -> [_ _ _ w935]
          tunnel: "Washer Water Temperature (60 ± 5°F):" -> [_ _ _ w934]
          tunnel: "Water Hardness (PPM):" -> [_ _ _ w933]
          tunnel: "Dryness Setting:" -> [_ _ _ w932]
          tunnel: "Dryer Type:" -> [_ _ _ w931]
          tunnel: "Exhaust:" -> [_ _ _ w930]
          tunnel: "Drying Cycle:" -> [_ _ _ w929]
          tunnel: "Cold Dryer Weigth" -> [_ _ _ w928]
          tunnel: "Load Type:" -> [_ _ _ w927]
          tunnel: "Nominal Load Weight (lbs):" -> [_ _ _ w926]
          tunnel: "Cycles Per Year" -> [_ _ _ w925]
          tunnel: "Moisture Reduction Factor" -> [_ _ _ w924]
          tunnel: "Field Use Factor" -> [_ _ _ w923]
          tunnel: "Energy Standard" -> [_ _ _ w922]
          frame "DOE Stand", "Portable Stand", Default {
          }
          frame "Dishwasher Kitchen" {
          }
          frame "HEWH", "PRAT", "HEWH RLT" {
          }
          frame "Dryer" {
            n520 = Bundle By Name(cluster=w937, "Washer Controls In.Initialize.Washer In.Appliance Details.Dryer.Dryer Initial IMC Data.Energy Standard"=w922, "Washer Controls In.Initialize.Washer In.Appliance Details.Dryer.Heat Setting:"=w935, "Washer Controls In.Initialize.Washer In.Appliance Details.Dryer.Washer Water Temperature (60 ± 5°F):"=w934, "Washer Controls In.Initialize.Washer In.Appliance Details.Dryer.Water Hardness (PPM):"=w933, "Washer Controls In.Initialize.Washer In.Appliance Details.Dryer.Dryness Setting:"=w932, "Washer Controls In.Initialize.Washer In.Appliance Details.Dryer.Dryer Type:"=w931, "Washer Controls In.Initialize.Washer In.Appliance Details.Dryer.Exhaust:"=w930, "Washer Controls In.Initialize.Washer In.Appliance Details.Dryer.Drying Cycle:"=w929, "Washer Controls In.Initialize.Washer In.Appliance Details.Dryer.Dryer Initial IMC Data.Empty Dryer Cold Weigth"=w928, "Washer Controls In.Initialize.Washer In.Appliance Details.Dryer.Load Type:"=w927, "Washer Controls In.Initialize.Washer In.Appliance Details.Dryer.Nominal Load Weight"=w926, "Washer Controls In.Initialize.Washer In.Appliance Details.Appliance Common.Cycles Per Year"=w925, "Washer Controls In.Initialize.Washer In.Appliance Details.Dryer.Dryer Initial IMC Data.Moisture Reduction Factor"=w924, "Washer Controls In.Initialize.Washer In.Appliance Details.Dryer.Dryer Initial IMC Data.Field Use Factor"=w923) -> (w936:T42)
          }
        }
        n521 = call <vilib>:"Add State(s) to Queue__jki_lib_state_machine.vi"("State(s) in (\"\")"=w915) -> ("States Out"=w918:string)  [unwired: 14 in]
      }
      frame "Get Refrigeration" {
        n522 = Unbundle By Name(w939) -> ("LV Program"=w938:T9)
        n523 = case shown="\"Refrigeration\"" w938 {
          tunnel: w939 -> [w944 w945 w946 w947 w948]
          tunnel: [w944 w945 w946 w947 w948] -> w941
          frame "DOE Stand", "Portable Stand", Default {
          }
          frame "Dishwasher Kitchen" {
          }
          frame "HEWH", "PRAT", "HEWH RLT" {
          }
          frame "Dryer" {
          }
          frame "Refrigeration" {
            # "Get Refrigeration specifics later"
          }
        }
        n524 = call <vilib>:"Add State(s) to Queue__jki_lib_state_machine.vi"("State(s) in (\"\")"=w940) -> ("States Out"=w943:string)  [unwired: 14 in]
      }
      frame "Generate Filename" {
        # "\"Create DIR & Filename \" VI references the \"Create Initial File\" VI 4 times\ncreating the Debug, INV, Current, and Bus Files. It also reference the \"Check Summary\"\nVI.  \n\nThe \"Create Initial File\" VI then references the \"Create Folder Location\", \"Create Initial\nFile Name\" VI, and \"Create Folder if Needed\" VI.  \n\n\"Create Folder Location\" VI takes in the File Locations & Lab ID & Station Label and\nconcatenates them all to create a folder.  This is also where the Date is added to the \nfolder name.\n\n\"Create Initial Filename\" VI takes in the folder locations and the washer info and creates a \nfilename which is then concatenated with the appropriate file type (.txt) and added to \nthe File Locations Out Cluster.  The \"Save Extract File Name\" file just bundles all the files\nto the file locations output.  The \"create file name\" VI simply concatenates the lab ID,\nTR Number, and Station ID to create the file name.  \n\nThere's also a \"Create Folder if Needed\" VI.  Didn't research that one much honestly"
        n525 = Unbundle By Name(w956) -> ("LV Program"=w954:T9, "Filepath In"=w955:T10, "Washer Controls In.Initialize.Washer In"=w953:T21)
        n526 = call "Save File Create Filename and Directories.vi"("LV Program"=w954, "Error In"=w950, "Initialize.Washer In"=w953, "File Paths In"=w955) -> ("Error Out"=w949:errorcluster, "Initialize.Washer Out"=w951:T21, "File Paths Out"=w952:T10)  [unwired: 5 in]
        n527 = Bundle By Name(cluster=w956, "Filepath In"=w952, "Washer Controls In.Initialize.Washer In"=w951) -> (w957:T42)
        n528 = call <vilib>:"Add State(s) to Queue__jki_lib_state_machine.vi"("State(s) in (\"\")"=w959) -> ("States Out"=w958:string)  [unwired: 14 in]
      }
      frame "Generate Header Data" {
        # "Check to make sure everything is\ncalibrated If its not, display a message\nto the user"
        n529 = Unbundle By Name(w968) -> ("Washer Controls In.Initialize.Washer In.Appliance Details"=w964:T22, "LV Program"=w963:T9, "Filepath In.General Setup Paths.Calibration File Path"=w962:path)
        n530 = call "Save File DOE Create Header File.vi"("Error In"=w961, "Calibration File Path"=w962, "LV Program"=w963, "Appliance Details"=w964) -> ("Error Out"=w960:errorcluster, "File Initialization Array"=w966:string[][])  [unwired: 6 in]
        n531 = Bundle By Name(cluster=w968, "Washer Controls In.Initialize.Washer In.Appliance Details.File Name Output Array"=w966) -> (w967:T42)
        n532 = call <vilib>:"Add State(s) to Queue__jki_lib_state_machine.vi"("State(s) in Front (\"\")"="Save Appliance Details" ("State(s) in Front (\"\")"), "State(s) in (\"\")"=w970) -> ("States Out"=w969:string)  [unwired: 13 in]
      }
      frame "Save Appliance Details" {
        # "This state allows us to use the \"read previous\" button"
        n533 = Unbundle By Name(w974) -> ("Filepath In"=w973:T10, "Washer Controls In.Initialize.Washer In.Appliance Details"=w977:T22, "Filepath In.General Setup Paths.File Save Previous Run Path"=w976:path)
        n534 = local write "Filepath In"(w973) -> ()
        n535 = call "Save File DOE Save Previous Input Data.vi"("State"=enum16{"Write", "Read"}."Write", "error in (no error)"=w972, "Appliance Previous Run Path"=w976, "Appliance Details"=w977) -> ("error out"=w971:errorcluster)  [unwired: 6 in, 1 out]
        n536 = call <vilib>:"Add State(s) to Queue__jki_lib_state_machine.vi"("State(s) in Front (\"\")"="Macro: Exit" ("State(s) in Front (\"\")"), "State(s) in (\"\")"=w980) -> ("States Out"=w979:string)  [unwired: 13 in]
      }
    }
    n537 = case shown="False" "Debug" {
      tunnel: w19 -> [w30 w33]
      tunnel: [w30 w32] -> w18
      tunnel: w17 -> [_ w31]
      frame False {
      }
      frame True {
        n538 = Build Array (concatenate)(w33, w31) -> (w32:string[])
        "States" <- w32
      }
    }
  }
  "error out" <- w9
  n539 = Unbundle By Name(w6) -> ("Washer Controls In"=→"Washer Controls Out":T12, "Filepath In"=→"Filepath Out":T10)
